vi "Main.vi"() -> ()   [LabVIEW 2019]
uses:
  States/TaskType.ctl
  States/Main_States.ctl
  States/Hand.ctl
  States/ROM_States.ctl
  Shared VIs/ClusterType/RobotStateType.ctl
  <vilib>/myRIO/Common/Instrument Driver Framework/myRIO v1.0/Encoder/typedefs/Encoder Signal Mode.ctl
  Shared VIs/Messages/NewPatientNotifierArgs.ctl
  Shared VIs/ModelSpecific/ETHMikeModel.ctl
  Shared VIs/ModelSpecific/ReadOnlyGlobalActions.ctl
  <vilib>/myRIO/Instrument Drivers/Onboard IO/AI/typedefs/AI Reference.ctl
  <vilib>/myRIO/Common/Instrument Driver Framework/Utilities/typedefs/myRIO Generic Hardware Reference.ctl
  <vilib>/myRIO/Common/Instrument Driver Framework/Utilities/typedefs/Hardware Version Enum.ctl
  <vilib>/myRIO/Common/Instrument Driver Framework/Utilities/typedefs/myRIO v1.0 Reference.ctl
  <vilib>/myRIO/Common/Instrument Driver Framework/Utilities/typedefs/Generic FPGA Reference.ctl
  <vilib>/myRIO/Common/Instrument Driver Framework/myRIO v1.0/AI/typedefs/AI Channels List.ctl
  <vilib>/myRIO/Common/Instrument Driver Framework/myRIO v1.0/AI/typedefs/AI Channels Enum.ctl
  <vilib>/myRIO/Common/Instrument Driver Framework/Utilities/typedefs/Analog Scaling Constants List.ctl
  <vilib>/myRIO/Common/Instrument Driver Framework/Utilities/typedefs/Analog Scaling Constants.ctl
  <vilib>/userDefined/High Color/nirio_resource_hc.ctl
  <vilib>/myRIO/Instrument Drivers/Onboard IO/AO/typedefs/AO Reference.ctl
  <vilib>/myRIO/Common/Instrument Driver Framework/myRIO v1.0/AO/typedefs/AO Channels List.ctl
  <vilib>/myRIO/Common/Instrument Driver Framework/myRIO v1.0/AO/typedefs/AO Channels Enum.ctl
  Shared VIs/ClusterType/TaskInfoType.ctl
  <vilib>/Platform/TimedLoop/XDataNode/timing_clust.ctl
  <vilib>/Platform/TimedLoop/XDataNode/nitl_modes.ctl
  <vilib>/Platform/TimedLoop/XDataNode/wakeup.ctl
  Shared VIs/Messages/UdpGlobalActions.ctl
  Shared VIs/TypeDef_TDMS_States.ctl
  Shared VIs/Messages/MsgHeader.ctl
  Shared VIs/Messages/PatientSelectMsg.ctl
  Shared VIs/Messages/CommandMsg.ctl
  Shared VIs/Messages/BackendInfoMsg.ctl
  <vilib>/myRIO/Common/Instrument Driver Framework/myRIO v1.0/AI/vis/myRIO v1.1 Open AI.vi
  <vilib>/myRIO/Common/Instrument Driver Framework/myRIO v1.0/AO/vis/myRIO v1.1 Open AO.vi
  <vilib>/myRIO/Common/Instrument Driver Framework/Utilities/vis/Validate Channels.vi
  <vilib>/myRIO/Common/Instrument Driver Framework/myRIO v1.0/AI/vis/myRIO v1.0 Reserve AI.vi
  <vilib>/myRIO/Common/Instrument Driver Framework/myRIO v1.0/AO/vis/myRIO v1.0 Reserve AO.vi
  <vilib>/myRIO/Common/Instrument Driver Framework/myRIO v1.0/AI/vis/myRIO v1.0 Close AI.vi
  <vilib>/myRIO/Common/Instrument Driver Framework/myRIO v1.0/Encoder/vis/myRIO v1.0 Close Encoder.vi
  <vilib>/myRIO/Common/Instrument Driver Framework/myRIO v1.0/AO/vis/myRIO v1.0 Close AO.vi
  <vilib>/myRIO/Common/Instrument Driver Framework/myRIO v1.0/AI/vis/myRIO v1.0 Build MUX Configuration AI.vi
  <vilib>/myRIO/Common/Instrument Driver Framework/myRIO v1.0/Resource Manager/vis/myRIO v1.0 Reserve Channel List.vi
  <vilib>/myRIO/Common/Instrument Driver Framework/myRIO v1.0/AO/vis/myRIO v1.0 Build MUX Configuration AO.vi
  <vilib>/myRIO/Common/Instrument Driver Framework/myRIO v1.0/AI/vis/myRIO v1.0 Unreserve AI.vi
  <vilib>/myRIO/Common/Instrument Driver Framework/myRIO v1.0/Encoder/vis/myRIO v1.0 Unreserve Encoder.vi
  <vilib>/myRIO/Common/Instrument Driver Framework/myRIO v1.0/AO/vis/myRIO v1.0 Unreserve AO.vi
  <vilib>/myRIO/Common/Instrument Driver Framework/myRIO v1.0/Resource Manager/vis/myRIO v1.0 Reserve Channel.vi
  <vilib>/myRIO/Common/Instrument Driver Framework/myRIO v1.0/Resource Manager/vis/myRIO v1.0 Unreserve Channel.vi
  <vilib>/myRIO/Common/Instrument Driver Framework/myRIO v1.0/Resource Manager/vis/myRIO v1.0 Unreserve Channel List.vi
  <vilib>/myRIO/Common/Instrument Driver Framework/myRIO v1.0/Encoder/vis/myRIO v1.0 Build MUX Configuration Encoder.vi
  <vilib>/myRIO/Common/Instrument Driver Framework/myRIO v1.0/Resource Manager/vis/myRIO v1.0 Build Mutex Name.vi
  <vilib>/myRIO/Common/Instrument Driver Framework/myRIO v1.0/Resource Manager/vis/myRIO v1.0 Create Configuration List.vi
  <vilib>/Utility/VariantDataType/GetNumericInfo.vi
  <vilib>/Utility/error.llb/Error Cluster From Error Code.vi
  <vilib>/myRIO/Common/Instrument Driver Framework/myRIO v1.0/myRIO v1.1 Open.vi
  <vilib>/myRIO/Common/Instrument Driver Framework/myRIO v1.0/AO/vis/myRIO v1.0 Get Scaling Constants AO.vi
  <vilib>/myRIO/Common/Instrument Driver Framework/Utilities/vis/IO Manager.vi
  <vilib>/myRIO/Common/Instrument Driver Framework/Utilities/vis/Configuration Manager.vi
  <vilib>/myRIO/Common/Instrument Driver Framework/myRIO v1.0/myRIO v1.0 Close.vi
  <vilib>/myRIO/Common/Instrument Driver Framework/myRIO v1.0/AO/vis/myRIO v1.0 Write AO.vi
  <vilib>/myRIO/Common/Instrument Driver Framework/myRIO v1.0/AI/vis/myRIO v1.0 Get Scaling Constants AI.vi
  <vilib>/functionblocks/Counter/Elapsed Timer/Elapsed Timer.vi
  <vilib>/myRIO/Common/Instrument Driver Framework/myRIO v1.0/Encoder/vis/myRIO v1.0 Enable Encoder.vi
  <vilib>/myRIO/Common/Instrument Driver Framework/myRIO v1.0/Encoder/vis/myRIO v1.0 Shutdown Encoder.vi
  <vilib>/myRIO/Common/Instrument Driver Framework/myRIO v1.0/Resource Manager/vis/myRIO v1.0 Configure IO.vi
  <vilib>/myRIO/Instrument Drivers/Onboard IO/AO/vis/myRIO AO Open.xnode
  <vilib>/myRIO/Instrument Drivers/Onboard IO/AI/vis/myRIO AI Open.xnode
  <vilib>/Platform/TimedLoop/XDataNode/XDataNode.xnode
  <vilib>/functionblocks/FB Core/FB Core.xnode
  <vilib>/myRIO/Instrument Drivers/Onboard IO/AO/AO.lvlib
  <vilib>/Platform/TimedLoop/XDataNode/XDNodeRunTimeDep.lvlib
  <vilib>/myRIO/Instrument Drivers/Onboard IO/Encoder/Encoder.lvlib
  <vilib>/myRIO/Instrument Drivers/Onboard IO/AI/AI.lvlib
  <vilib>/functionblocks/NI_FunctionBlock Libraries.lvlib
  <vilib>/addons/control/pid/NI_PID_pid.lvlib
  <vilib>/ptbypt/NI_PtbyPt.lvlib
panel:
  out "start value":dbl
  out "Haptic Bump Force Frontend [N]":dbl
  out "difference at start":dbl
  out "Direction":i32
  out "Haptic Bump Force [N]":dbl format="%#_13g"
  out "Plateau length [deg]":dbl
  out "Ramp length [deg]":dbl=4.0 format="%#_13g"
  out "Starting Position Frontend [deg]":dbl
  out "Target Position Frontend [deg]":dbl
  out "RobotState":T1
  out "SkipSignal":bool
  out "Force_calib_value":dbl
  out "Velocity_calib_value":dbl
  out "LogFileOpen":bool
  out "Phase Trial Count":i16
  out "Error which lead\nto TCP close":errorcluster
  out "TCP Error":errorcluster
  out "UDP Error":errorcluster
  in  "stop":bool
  out "SelectedHand":T2
  out "Connected":bool
  out "Remote IP":u32 format="%x"
  out "StopRequested":bool
  in  "TCP Server Port":u16=6662
  in  "UDP Destination Port":u16=6661
  out "DateTime":string
  out "SubjectNr":string
  out "StopSignal":bool
  out "RestartSignal":bool
  out "StartSignal":bool
  out "FrontendStartedSignal":bool
  out "Flexion":bool
  out "TaskFinished":bool
  out "ROM State":T3=enum."Passive"
  out "LeftHand":bool
  out "Machine State":T4=enum."StartTrial"
  out "MovingToTarget":bool=TRUE
  out "ROM max":dbl
  out "ROM min":dbl
  out "Zero Position":dbl
  out "Largest USB Partition Path":path
  out "Trial Nr":i16
  out "Starting position":dbl
  out "Target Array":dbl[](array[numeric])
  out "TaskType":T5
  out "Current Setpoint [A]":dbl
  out "Finished late?":bool
  out "Target state?":bool
  out "Target Position [deg]":dbl
  # "Frontend Connection"
  # "Command Signals"
  # "Robot State"
  # "Patient Data"
  # "Task State"
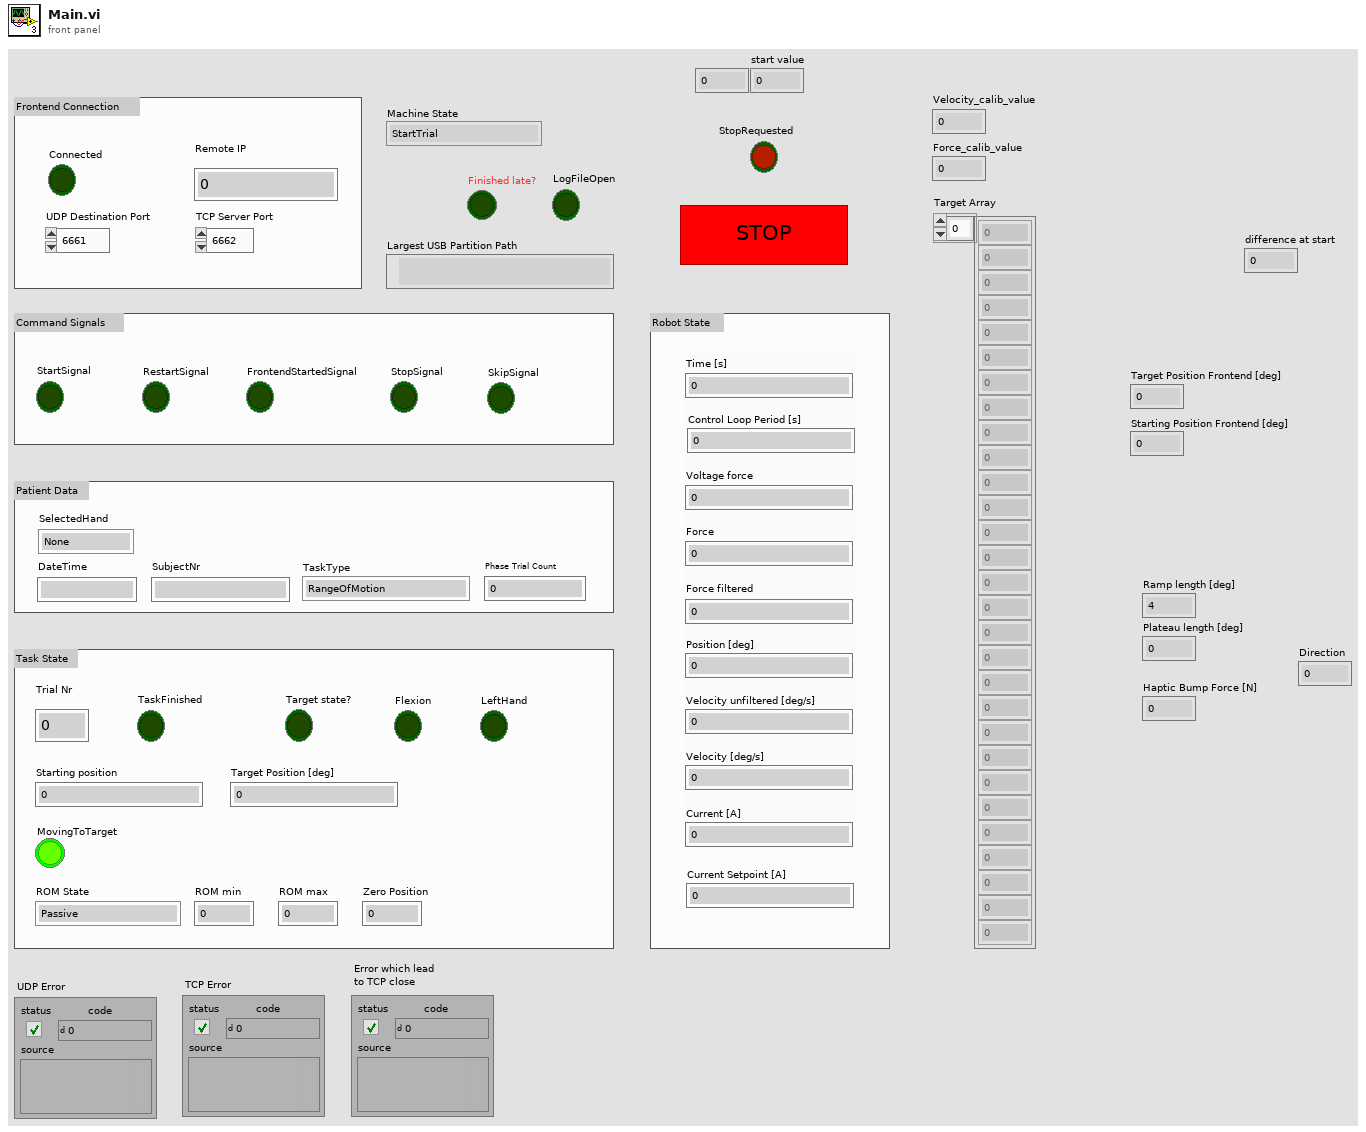
[diagram p1: front panel]
types:
  T1 = typedef "RobotStateType.ctl" = cluster{"Time [s]":dbl, "Voltage force":dbl, "Force":dbl, "Force filtered":dbl, "Position [deg]":dbl, "Velocity unfiltered [deg/s]":dbl, "Velocity [deg/s]":dbl, "Current [A]":dbl, "Control Loop Period [s]":dbl}
  T2 = typedef "Hand.ctl" = enum8{"None", "Left", "Right"}
  T3 = typedef "ROM_States.ctl" = enum8{"Active", "Passive", "AutomaticPassive"}
  T4 = typedef "Main_States.ctl" = enum16{"Hand choice", "StartTask", "StartTrial", "Show target", "Resetting", "WaitingForRestart"}
  T5 = typedef "TaskType.ctl" = enum8{"RangeOfMotion", "Force", "Motor", "Sensorimotor", "PositionMatching", "PreciseReaching", "PassiveMatching", "ActiveMatching", "TeachAndReproduce", "HapticBump"}
  T6 = typedef "NewPatientNotifierArgs.ctl" = cluster{"Left":bool, "Mode":T5, "Name":string, "Timestamp":string, "StudyName":string}
  T7 = cluster{"read mode":enum16{"polling", "blocking"}, "write mode":enum16{"polling", "blocking"}}
  T8 = typedef "nirio_resource_hc.ctl" = tag
  T9 = typedef "Hardware Version Enum.ctl" = enum16{"Unknown", "myRIO-1900", "myRIO-1950", "roboRIO", "NI ELVIS RIO CM", "ELVIS III"}
  T10 = typedef "TypeDef_TDMS_States.ctl" = enum16{"WaitingForCreate", "Create", "Buffering", "Flushing", "Write", "Close"}
  T11 = enum16{"open", "open or create", "create or replace", "create", "open (read-only)"}
  T12 = typedef "XDNodeRunTimeDep.lvlib/timing_clust.ctl" = cluster{"Expected End [f-1]":u64, "Actual End [f-1]":u64, "Finished Late? [f-1]":bool, "Expected End [i-1]":u64, "Actual End [i-1]":u64, "Finished Late? [i-1]":bool, "Expected Start [i]":u64, "Actual Start [i]":u64, "Expected Start [f]":u64, "Actual Start [f]":u64, "Source Name":string, "Structure Name":string, "Period":i64, "Deadline":i64, "Offset":i64, "Start":i64, "Priority":i32, "Timeout":i32, "Mode":T13, "Wakeup Reason":T14, "Error":errorcluster, "Source Type":string, "Secondary Source Type":string, "Global End Time":u64, "Global Start Time":u64, "Frame Duration":u64, "Iteration Duration":u64, "Assigned CPU":i32, "I/O Scan Engine Mode":u32}
  T13 = typedef "XDNodeRunTimeDep.lvlib/nitl_modes.ctl" = enum32{"No Change", "Process missed periods, maintain original phase", "Discard missed periods, maintain original phase", "Process missed periods, ignore original phase", "Discard missed periods, ignore original phase"}
  T14 = typedef "XDNodeRunTimeDep.lvlib/wakeup.ctl" = enum32{"Normal", "Aborted", "Asynchronous wakeup", "Timing source error", "Timed loop error", "Timeout"}
  T15 = enum8{"Invalid", "PatientSelect", "Command", "Skip", "BackendInfoReq", "UnknownOp (Must be Last)"}
  T16 = typedef "MsgHeader.ctl" = cluster{"MsgType [0]":u8, "MsgLen [1:2]":u16}
  T17 = typedef "PatientSelectMsg.ctl" = cluster{"LeftHand":bool, "AssessmentMode":u8, "SubjectNr":string, "DateTime":string, "PhaseTrialCount":i32, "StudyName":string}
  T18 = typedef "CommandMsg.ctl" = cluster{"EmergencyStop":bool, "Start":bool, "Restart":bool, "FrontendStarted":bool, "Close":bool, "StartingPosition":sgl, "TargetPosition":sgl, "HapticBumpForce":dbl}
  T19 = typedef "BackendInfoMsg.ctl" = cluster{"ProtocolVersion":u16, "DataPath":string}
  T20 = typedef "UdpGlobalActions.ctl" = enum16{"Read", "Write"}
  T21 = typedef "ReadOnlyGlobalActions.ctl" = enum16{"Initialize", "Read", "Write"}
  T22 = typedef "ETHMikeModel.ctl" = enum16{"ETH Mike #1", "ETH Mike #2", "ETH Mike #3", "ETH Mike #4", "ETH MIKE #5"}
  T23 = typedef "Encoder Signal Mode.ctl" = enum16{"Quadrature phase signal", "Step and direction signal"}
  T24 = typedef "AO.lvlib/AO Reference.ctl" = cluster{"myRIO Reference":T25, "AO Channel List":T28, "AO Scaling Constant List":T30}
  T25 = typedef "myRIO Generic Hardware Reference.ctl" = cluster{"myRIO Model":T9, "myRIO Hardware Reference":T26}
  T26 = typedef "myRIO v1.0 Reference.ctl" = cluster{"Generic FPGA Reference":T27, "Allow multiple opens":bool}
  T27 = typedef "Generic FPGA Reference.ctl" = refnum<k20>
  T28 = typedef "AO Channels List.ctl" = T29[]
  T29 = typedef "AO Channels Enum.ctl" = enum16{"Not Connected", "AudioOut/Left", "AudioOut/Right", "C/AO0", "C/AO1", "A/AO0", "A/AO1", "B/AO0", "B/AO1"}
  T30 = typedef "Analog Scaling Constants List.ctl" = T31[]
  T31 = typedef "Analog Scaling Constants.ctl" = cluster{"LSB Weight (Volts)":dbl, "Offset (Volts)":dbl, "Signed?":bool}
  T32 = typedef "Encoder.lvlib/Encoder Reference.ctl" = cluster{"myRIO Reference":T25, "Encoder Channels Enum":T33}
  T33 = typedef "Encoder Channels Enum.ctl" = enum16{"Not Connected", "C/ENC0", "C/ENC1", "A/ENC", "A/ENC0", "A/ENC1", "A/ENC2", "A/ENC3", "A/ENC4", "A/ENC5", "A/ENC6", "A/ENC7", "A/ENC8", "A/ENC9", "B/ENC", "B/ENC0", "B/ENC1", "B/ENC2", "B/ENC3", "B/ENC4", "B/ENC5", "B/ENC6", "B/ENC7", "B/ENC8", "B/ENC9", "DIO/ENC0", "DIO/ENC1", "DIO/ENC2", "DIO/ENC3", "DIO/ENC4"}
  T34 = typedef "AI.lvlib/AI Reference.ctl" = cluster{"myRIO Reference":T25, "AI Channels List":T35, "AI Scaling Constants List":T30}
  T35 = typedef "AI Channels List.ctl" = T36[]
  T36 = typedef "AI Channels Enum.ctl" = enum16{"Not Connected", "AudioIn/Left", "AudioIn/Right", "C/AI0", "C/AI1", "A/AI0", "A/AI1", "A/AI2", "A/AI3", "A/AI4", "A/AI5", "A/AI6", "A/AI7", "B/AI0", "B/AI1", "B/AI2", "B/AI3", "B/AI4", "B/AI5", "B/AI6", "B/AI7", "AI/AI0", "AI/AI1", "AI/AI2", "AI/AI3", "A/AI0 (DIFF)", "A/AI1 (DIFF)", "A/AI2 (DIFF)", "A/AI3 (DIFF)", "B/AI0 (DIFF)", "B/AI1 (DIFF)", "B/AI2 (DIFF)", "B/AI3 (DIFF)"}
  T37 = cluster{"Encoder":T32, "Tachometer":T34, "Motor Current Monitor":T34, "Force Sensor":T34}
  T38 = typedef "LVAllMonitorsDisplayTypeDef.ctl" = cluster{"Bounds":cluster{"Left":i16, "Top":i16, "Right":i16, "Bottom":i16}, "Depth":i16}[]
  T39 = cluster{"Bounds":cluster{"Left":i16, "Top":i16, "Right":i16, "Bottom":i16}, "Depth":i16}
  T40 = cluster{"Left":i16, "Top":i16, "Right":i16, "Bottom":i16}
  T41 = typedef "TaskInfoType.ctl" = cluster{"Task Type":T5, "Phase Trial Count":i16, "Left Hand":bool}
  T42 = enum16{"Standard", "Buffered", "CRLF", "Immediate"}
  T43 = typedef "UDPRobotState.ctl" = cluster{"Counter":u32, "Time":sgl, "Position":sgl, "StartingPosition":sgl, "TargetPosition":sgl, "Force":sgl, "TrialNr":u8, "RomState":u8, "TargetState":bool, "Finished":bool, "Flexion":bool}
  T44 = typedef "PID_Settings.ctl" = cluster{"Gains":T45, "Non-linear gain":T46, "D-Part variable":T48, "Velocity estimate dy/dt":T49, "Anti reset windup":bool, "I-Part error band":dbl, "Output range":T50}
  T45 = typedef "Gains.ctl" = cluster{"K(e)":dbl, "Kp":dbl, "Ki":dbl, "Kd":dbl}
  T46 = typedef "NonLinearGainParams.ctl" = cluster{"Non-linear gain P":T47, "Non-linear gain I":T47, "Non-linear gain D":T47}
  T47 = typedef "NonLinearGain.ctl" = enum16{"exponential", "quadratic", "off"}
  T48 = typedef "DPartVariable.ctl" = enum16{"error", "process variable"}
  T49 = typedef "VelocityEstimate.ctl" = enum16{"derivative", "external"}
  T50 = typedef "OutputRange.ctl" = cluster{"output high":dbl, "output low":dbl}
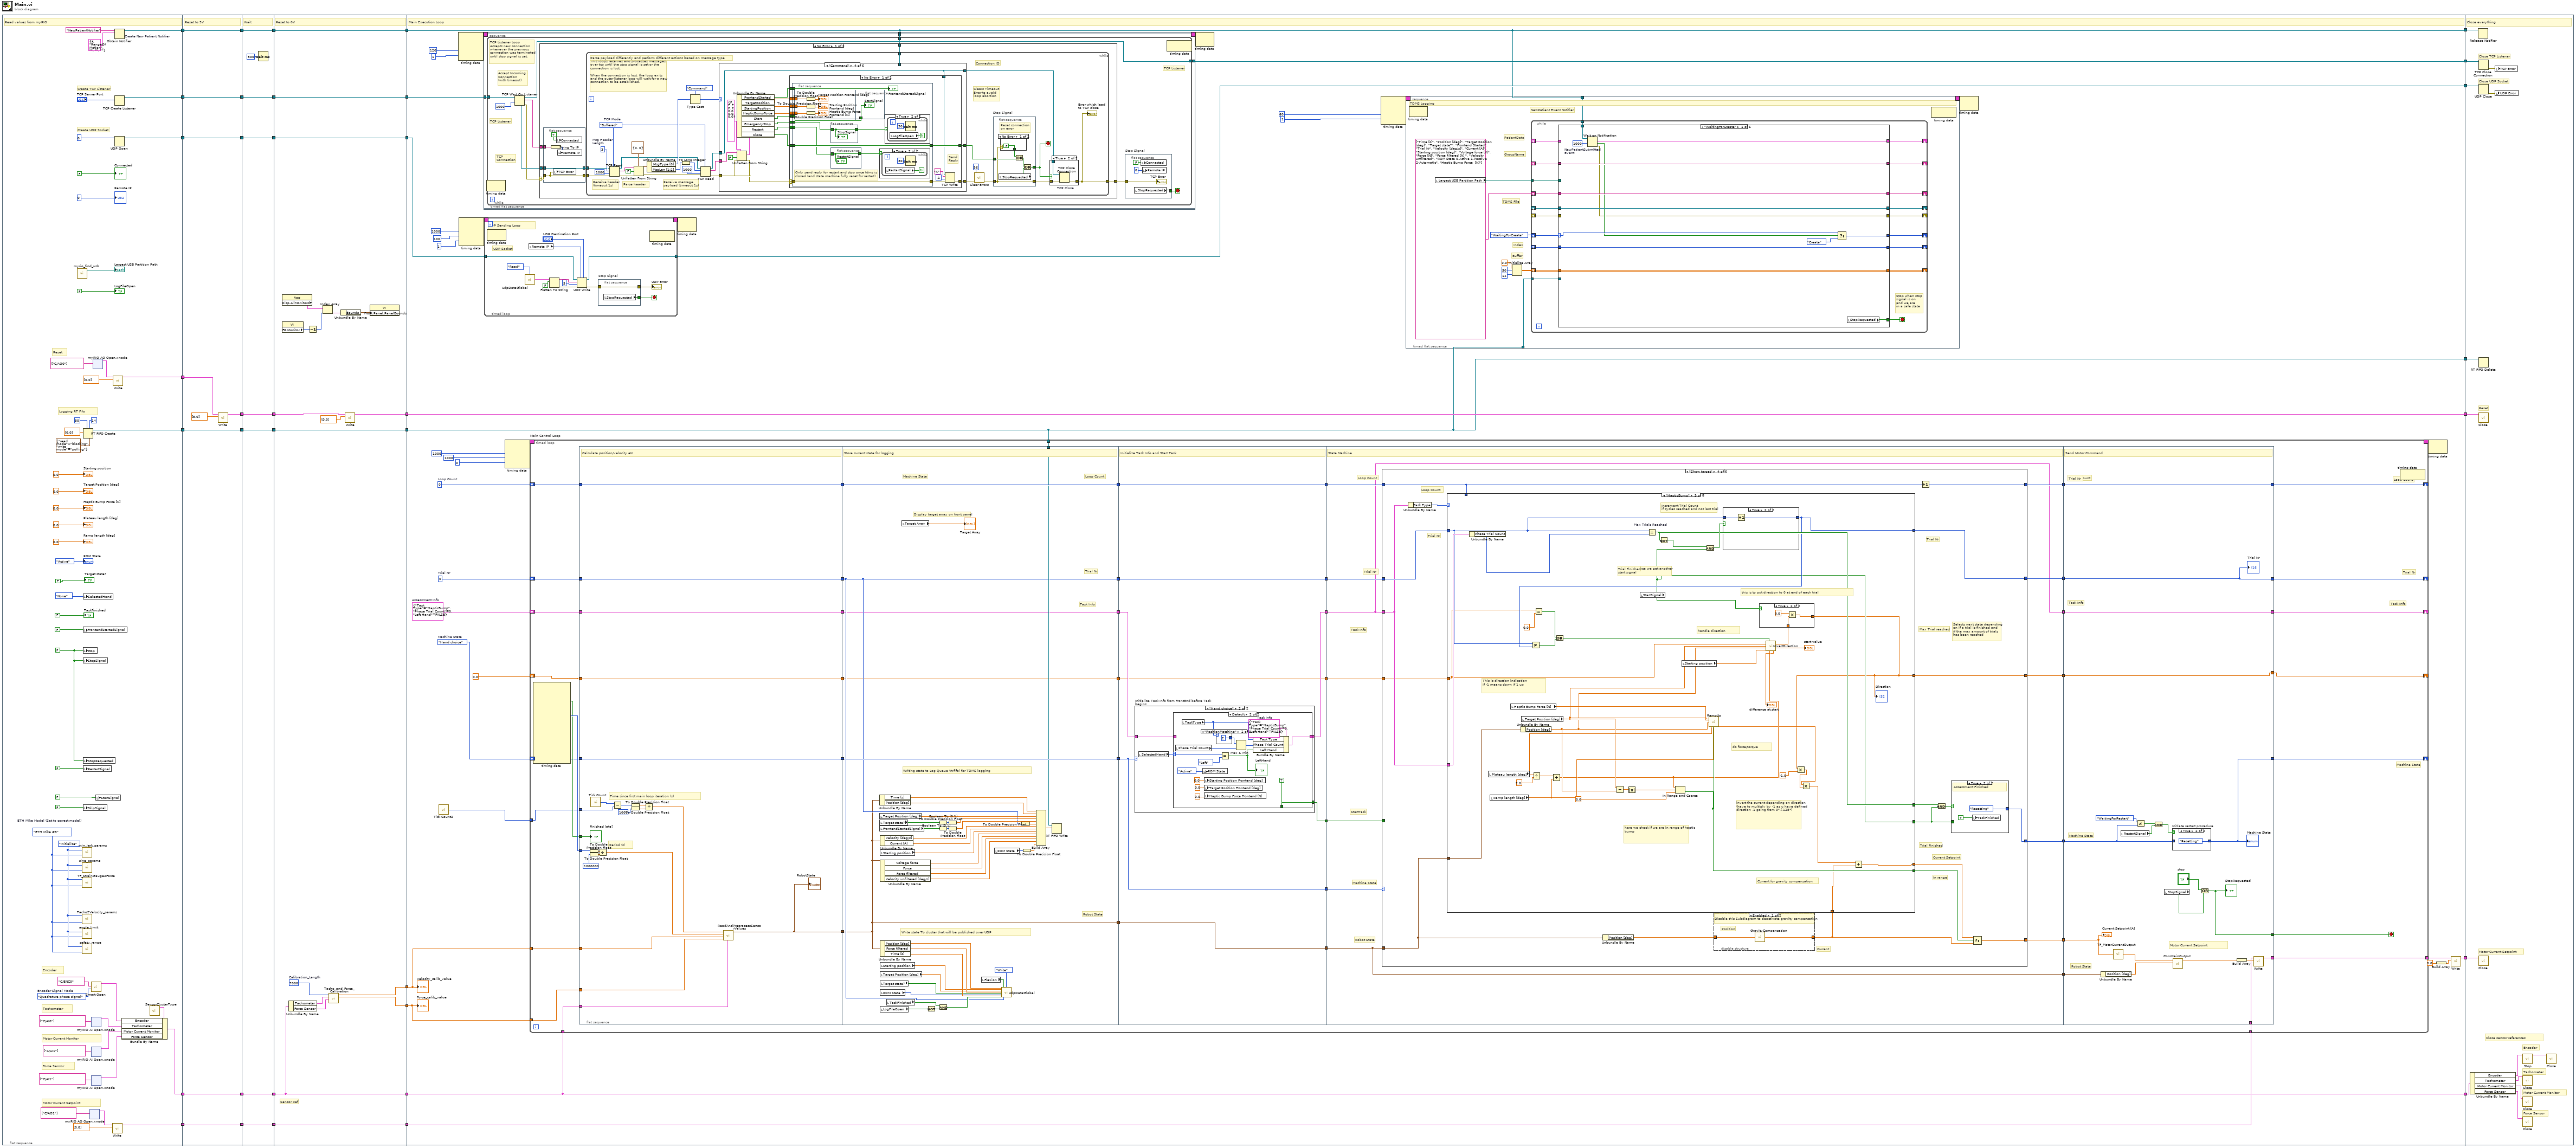
[diagram p0: block diagram]
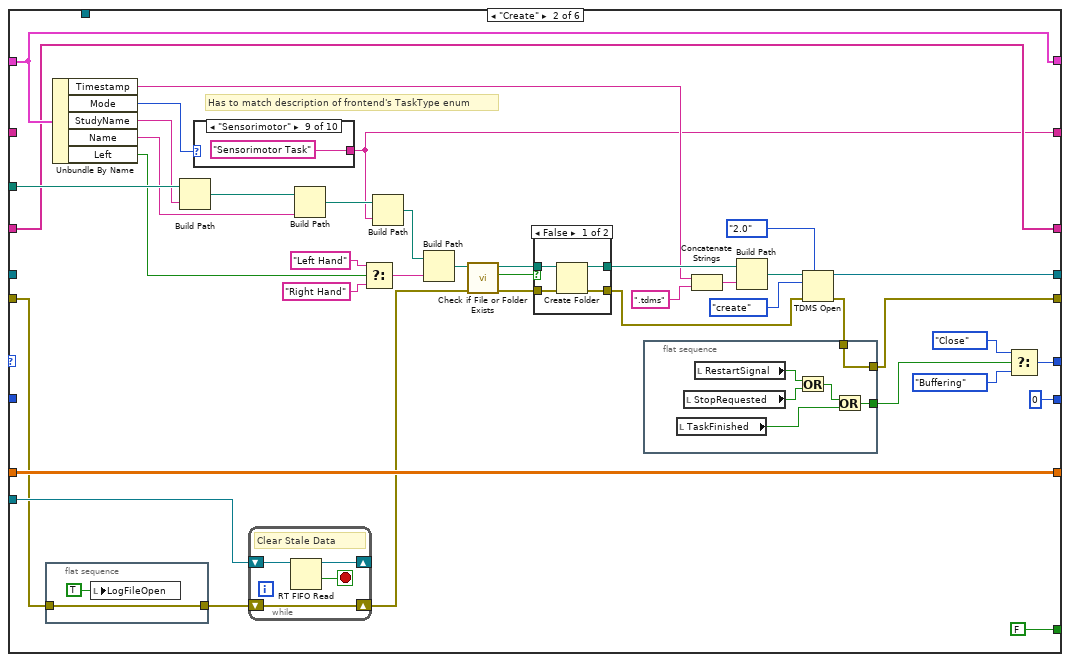
[diagram p2: hidden frame]
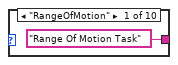
[diagram p4: hidden frame]
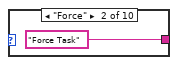
[diagram p5: hidden frame]
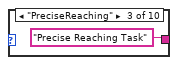
[diagram p6: hidden frame]
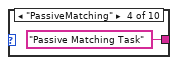
[diagram p7: hidden frame]
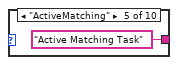
[diagram p8: hidden frame]
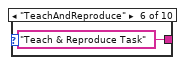
[diagram p9: hidden frame]
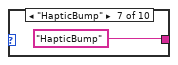
[diagram p10: hidden frame]
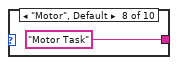
[diagram p11: hidden frame]
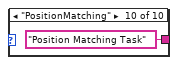
[diagram p12: hidden frame]
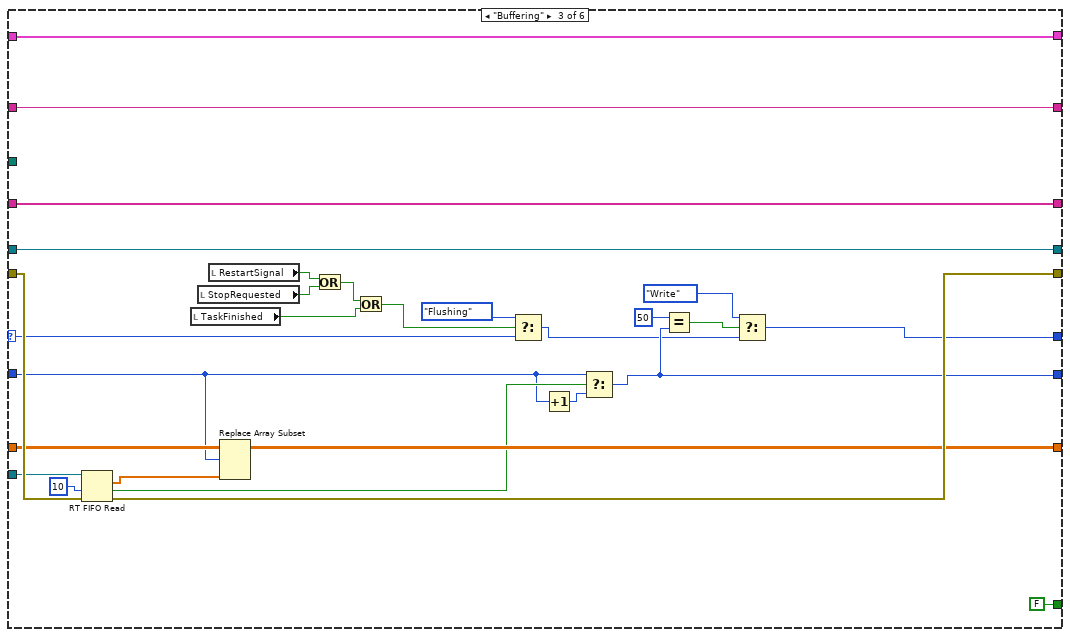
[diagram p13: hidden frame]
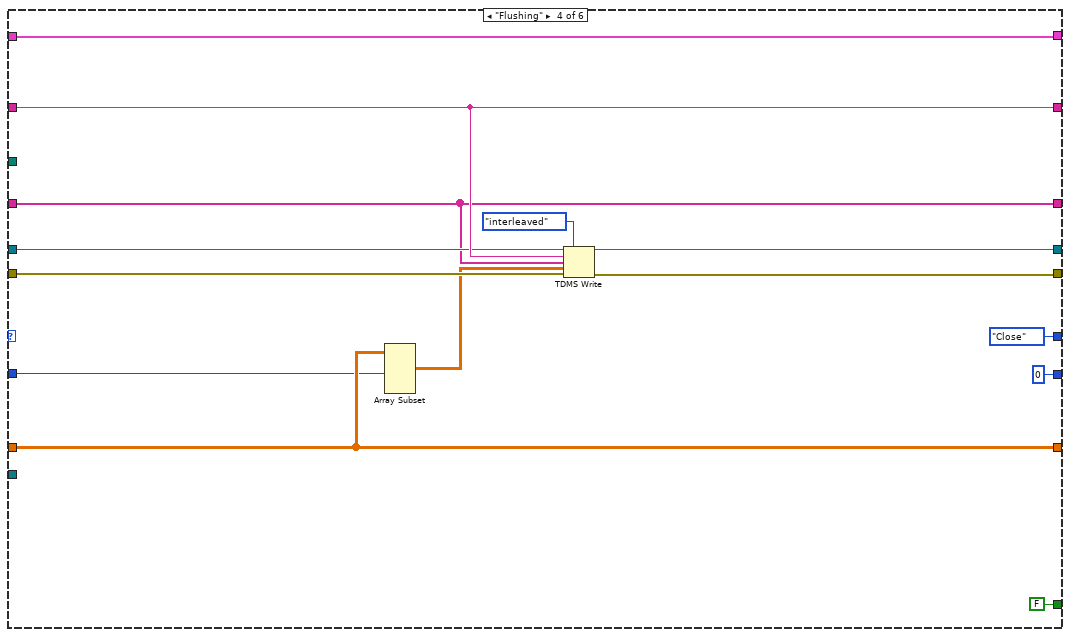
[diagram p14: hidden frame]
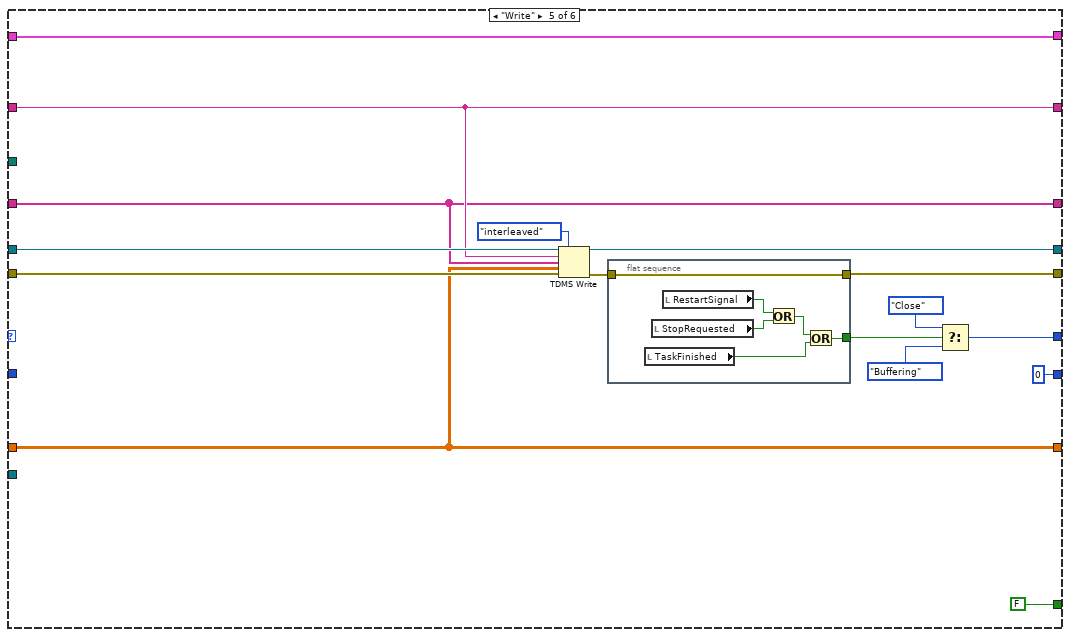
[diagram p15: hidden frame]
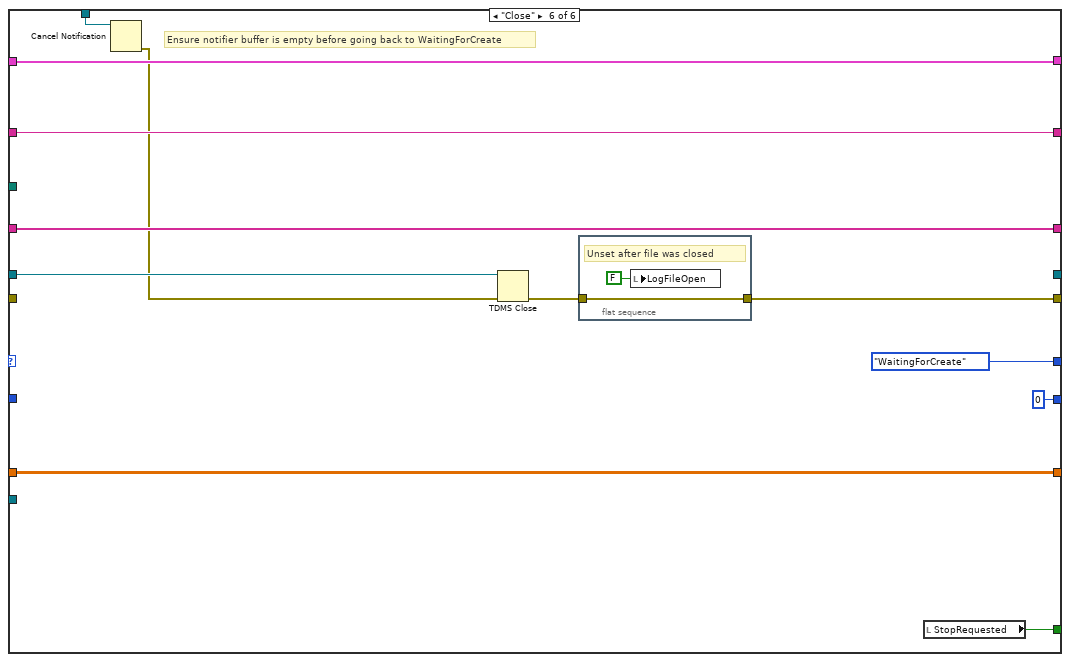
[diagram p16: hidden frame]
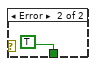
[diagram p18: hidden frame]
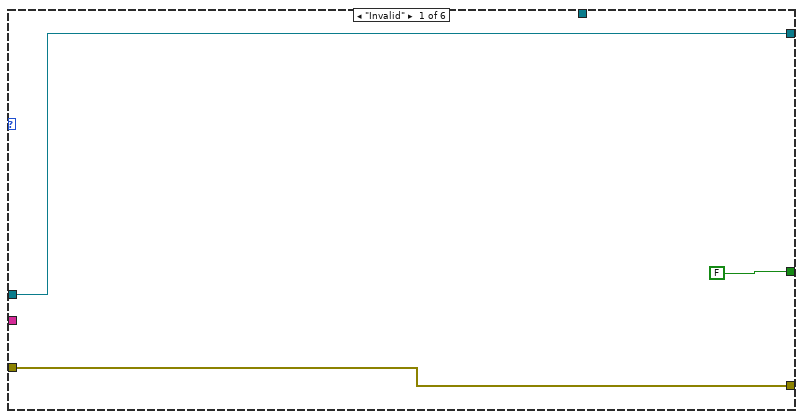
[diagram p19: hidden frame]
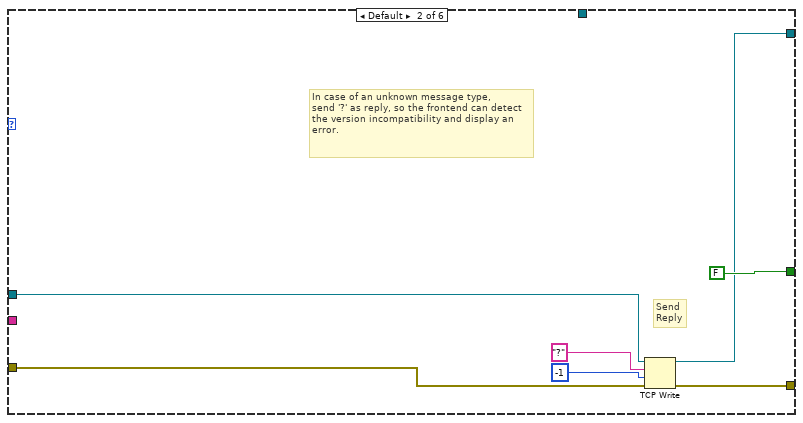
[diagram p20: hidden frame]
diagram:
  n1 = flat-sequence {
    tunnel: [w78] -> w37
    tunnel: [w69] -> w28
    tunnel: [w67] -> w24
    tunnel: [w56] -> w18
    tunnel: [w55] -> w14
    tunnel: [w42] -> w7
    tunnel: [w41] -> w1
    tunnel: w37 -> [w186]
    tunnel: [w185] -> w36
    tunnel: [w184] -> w29
    tunnel: w28 -> [w184]
    tunnel: [w183] -> w25
    tunnel: w24 -> [w183]
    tunnel: [w182] -> w19
    tunnel: w18 -> [w182]
    tunnel: [w181] -> w15
    tunnel: w14 -> [w181]
    tunnel: [w180] -> w8
    tunnel: w7 -> [w180]
    tunnel: [w179] -> w2
    tunnel: w1 -> [w179]
    tunnel: w36 -> [w194]
    tunnel: [w194] -> w35
    tunnel: [w193] -> w30
    tunnel: w29 -> [w193]
    tunnel: [w192] -> w26
    tunnel: w25 -> [w192]
    tunnel: [w191] -> w20
    tunnel: w19 -> [w191]
    tunnel: [w190] -> w16
    tunnel: w15 -> [w190]
    tunnel: [w189] -> w9
    tunnel: w8 -> [w189]
    tunnel: [w188] -> w3
    tunnel: w2 -> [w188]
    tunnel: w35 -> [w213]
    tunnel: [w212] -> w34
    tunnel: [w206] -> w31
    tunnel: w30 -> [w206]
    tunnel: w26 -> [w205]
    tunnel: [w205] -> w23
    tunnel: [w204] -> w21
    tunnel: w20 -> [w204]
    tunnel: [w203] -> w17
    tunnel: w16 -> [w203]
    tunnel: [w201] -> w11
    tunnel: [w200] -> w10
    tunnel: w9 -> [w197]
    tunnel: [w197] -> w6
    tunnel: [w196] -> w4
    tunnel: w3 -> [w196]
    tunnel: w34 -> [w251]
    tunnel: [w225] -> w33
    tunnel: [w251] -> w32
    tunnel: w31 -> [w244]
    tunnel: [w234] -> w27
    tunnel: w23 -> [w243]
    tunnel: [w233] -> w22
    tunnel: w21 -> [w219]
    tunnel: w17 -> [w227]
    tunnel: [w227] -> w13
    tunnel: [w219] -> w12
    tunnel: w11 -> [w216]
    tunnel: w10 -> [w222]
    tunnel: w6 -> [w221]
    tunnel: [w221] -> w5
    tunnel: w4 -> [w217]
    tunnel: w33 -> [w1526]
    tunnel: w32 -> [w1533]
    tunnel: w27 -> [w1532]
    tunnel: w22 -> [w1531]
    tunnel: w13 -> [w1528]
    tunnel: w12 -> [w1527]
    tunnel: w5 -> [w1525]
    frame #0 {
      w49 = ReadOnlyGlobalActions."Initialize" ("Action (Read)")
      w48 = ETHMikeModel."ETH Mike #3"  # ETH Mike Model (Set to correct model)
      w63 = FALSE ("stop")
      w84 = Encoder_Signal_Mode."Quadrature phase signal"  # Encoder Signal Mode
      # "Logging RT Fifo"
      # "Create TCP Listener"
      # "Create UDP Socket"
      # "Force Sensor"
      # "Tachometer"
      # "Motor Current Monitor"
      # "Motor Current Setpoint"
      # "Reset"
      # "Encoder"
      # "Read values from myRIO"
      n2 = call "myrio_find_usb.vi"() -> ("Largest USB Partition Path"=→"Largest USB Partition Path":path)  [unwired: 9 in, 2 out]
      n3 = call "min_jerk_params.vi"("Action (Read)"=w49, "ETH Mike Model"=w48) -> ()  [unwired: 17 in, 1 out]
      n4 = call "sine_params.vi"("Action (Read)"=w49, "ETH Mike Model"=w48) -> ()  [unwired: 17 in, 1 out]
      n5 = call "TF_StrainGauge2Force.vi"("Action (Read)"=w49, "ETH Mike Model"=w48) -> ()  [unwired: 3 in, 1 out]
      n6 = call "Tacho2Velocity_params.vi"("Action (Read)"=w49, "ETH Mike Model"=w48) -> ()  [unwired: 3 in, 1 out]
      n7 = call "angle_limit.vi"("ETH Mike Model"=w48, "Action (Read)"=w49) -> ()  [unwired: 1 out]
      n8 = call "safety_range.vi"("ETH Mike Model"=w48, "Action (Read)"=w49) -> ()  [unwired: 1 out]
      n9 = RT FIFO Create(1:dbl[] [0.0] ("Values"), 4:u32 50 ("size (10)"), 6:u32 14 ("elements in array (1)"), 7:T7 {"read mode"=enum."blocking", "write mode"=enum."polling"} ("r/w modes (polling,polling)")) -> (8:w56:refnum<k33>)  [unwired: 4 in, 2 out]
      n10 = local write "SelectedHand"(Hand."None" ("Enum")) -> ()
      n11 = local write "FrontendStartedSignal"(FALSE) -> ()
      n12 = local write "stop"(w63) -> ()
      n13 = local write "StopSignal"(w63) -> ()
      n14 = local write "StopRequested"(w63) -> ()
      n15 = local write "RestartSignal"(FALSE ("Restart")) -> ()
      n16 = local write "SkipSignal"(FALSE ("StartSignal")) -> ()
      n17 = xnode "myRIO AO Open.xnode"("Channel Names"=tag[] ["C/AO1"]) -> ("AO Ref Out"=w82:T24)  [unwired: 2 in, 1 out]
      n18 = call <vilib>:"Smart Open.vi"("Encoder Signal Mode"=w84, "Channel Name"=tag "C/ENC0") -> ("Encoder Ref Out"=w46:T32)  [unwired: 8 in, 1 out]
      n19 = xnode "myRIO AI Open.xnode"("Channel Names"=tag[] ["C/AI0"]) -> ("AI Ref Out"=w45:T34)  [unwired: 2 in, 1 out]
      n20 = xnode "myRIO AI Open.xnode"("Channel Names"=tag[] ["A/AI1"]) -> ("AI Ref Out"=w44:T34)  [unwired: 2 in, 1 out]
      n21 = xnode "myRIO AI Open.xnode"("Channel Names"=tag[] ["C/AI1"]) -> ("AI Ref Out"=w43:T34)  [unwired: 2 in, 1 out]
      n22 = xnode "myRIO AO Open.xnode"("Channel Names"=tag[] ["C/AO0"]) -> ("AO Ref Out"=w87:T24)  [unwired: 2 in, 1 out]
      n23 = local write "StartSignal"(FALSE ("StartSignal")) -> ()
      n24 = call <vilib>:"Write.vi"("Values"=dbl[] [0.0], "AO Ref In"=w82) -> ("AO Ref Out"=w41:T24)  [unwired: 7 in, 1 out]
      n25 = call <vilib>:"Write.vi"("Values"=dbl[] [0.0], "AO Ref In"=w87) -> ("AO Ref Out"=w78:T24)  [unwired: 7 in, 1 out]
      n26 = Obtain Notifier "Create New Patient Notifier"(name (unnamed)="NewPatientNotifier", notification data type=T6 {"Left"=FALSE, "Mode"=enum."RangeOfMotion", "Name"="", "Timestamp"="", "StudyName"=""}) -> (notifier out=w55:refnum<notifier>)  [unwired: 2 in, 2 out]
      n27 = TCP Create Listener(10:"TCP Server Port") -> (3:w67:refnum<k5>)  [unwired: 4 in, 2 out]
      n28 = UDP Open(11:u16 0) -> (port=w69:refnum<k16>)  [unwired: 4 in, 2 out]
      n29 = call "SensorClusterType.vi"() -> ("Cluster"=w47:T37)  [unwired: 11 in]
      n30 = Bundle By Name(cluster=w47, "Encoder"=w46, "Tachometer"=w45, "Motor Current Monitor"=w44, "Force Sensor"=w43) -> (w42:T37)
      "Target state?" <- FALSE ("Target state?")
      "Target Position [deg]" <- 0.0 ("Target Position [deg]")
      "ROM State" <- ROM_States."Active" ("Enum")
      "Connected" <- FALSE
      "Remote IP" <- u32 0
      "LogFileOpen" <- FALSE ("LogFileOpen")
      "TaskFinished" <- FALSE ("AssessmentFinished")
      "Starting position" <- 0.0 ("Starting position")
      "Ramp length [deg]" <- 0.0
      "Plateau length [deg]" <- 0.0 ("Target Position [deg]")
      "Haptic Bump Force [N]" <- 0.0
    }
    frame #1 {
      # "Reset to 5V"
      n31 = call <vilib>:"Write.vi"("Values"=dbl[] [5.0], "AO Ref In"=w186) -> ("AO Ref Out"=w185:T24)  [unwired: 7 in, 1 out]
    }
    frame #2 {
      # "Wait"
      n32 = Wait (ms)(milliseconds to wait=u32 500) -> ()  [unwired: 1 out]
    }
    frame #3 {
      w202 = 7000  # Calibration_Length
      # "Sensor Ref"
      # "Reset to 0V"
      n33 = property class="App"() -> ("Disp.AllMonitors"=w211:T38)  [unwired: 2 in, 2 out]
      n34 = property class="VI"() -> ("FP.Monitor"=w210:u16)  [unwired: 2 in, 2 out]
      n35 = Unbundle By Name(w197) -> ("Tachometer"=w199:T34, "Force Sensor"=w198:T34)
      n36 = Decrement(x=w210) -> (x-1=w209:u16)
      n37 = Index Array(array=w211, index=w209) -> (element=w208:T39)
      n38 = call "Tacho_and_Force_Calibration.vi"("Force Ref In"=w198, "Tacho Ref In"=w199, "Calibration_Length"=w202) -> ("Force_calib_value"=w200:dbl, "Velocity_calib_value"=w201:dbl)  [unwired: 7 in]
      n39 = Unbundle By Name(w208) -> ("Bounds"=w207:T40)
      n40 = call <vilib>:"Write.vi"("Values"=dbl[] [0.0], "AO Ref In"=w213) -> ("AO Ref Out"=w212:T24)  [unwired: 7 in, 1 out]
      n41 = property class="VI"("Front Panel.PanelBounds"=w207) -> ()  [unwired: 2 in, 2 out]
    }
    frame #4 {
      w218 = T41 {"Task Type"=enum."HapticBump", "Phase Trial Count"=0, "Left Hand"=FALSE}  # Assessment Info
      w247 = i16 0  # Trial Nr
      w248 = Main_States."Hand choice"  # Machine State
      w232 = 0  # Loop Count
      # "Main Execution Loop"
      n42 = call "Tick Count2"() -> ("Tick Count(mSec)"=w220:u32)
      n43 = node-c288(120 ("Priority"), 1 ("Processor")) -> (w240:T12)  [unwired: 2 in]
      n44 = node-c288(i64 1000 ("Period"), 100 ("Priority"), 1 ("Processor")) -> (w246:T12)  [unwired: 1 in]
      n45 = timed-sequence {
        timing: w240 -> [_]
        timing-out: [_] -> w239
        tunnel: w243 -> [w453]
        tunnel: [w452] -> w233
        tunnel: w227 -> [w451]
        n46 = timed-flat-sequence {
          tunnel: w453 -> [w456]
          tunnel: [w455] -> w452
          tunnel: w451 -> [w454]
          n47 = node-c288() -> ()  [unwired: 1 in, 1 out]
          n48 = while {
            tunnel: w456 -> [w467]
            tunnel: [w460] -> w455
            tunnel: w454 -> [w459]
            stop <- w462 stop-if-true
            # "TCP Listener"
            # "TCP Listener"
            # "TCP \nConnection"
            # "TCP Listener Loop\nAccepts new connection\nwhenever the previous\nconnection was terminated\nuntil stop signal is set."
            # "Accept Incoming\nConnection\n(with timeout)"
            n49 = TCP Wait On Listener ("TCP Accept")(9:1000, 11:w467) -> (0:w465:errorcluster, 2:w461:string, 3:w460:refnum<k5>, 4:w466:refnum<k5>)  [unwired: 2 in, 1 out]
            n50 = case shown="No Error" w465 {
              selector: w465 -> [w477 w669]
              tunnel: w466 -> [w475 _]
              tunnel: [w478 w669] -> w463
              tunnel: w461 -> [w473 _]
              tunnel: w459 -> [w472 _]
              frame No Error {
                n51 = flat-sequence {
                  tunnel: w477 -> [w479]
                  tunnel: [w479] -> w476
                  tunnel: w475 -> [w481]
                  tunnel: [w481] -> w474
                  tunnel: w473 -> [w480]
                  frame #0 {
                    n52 = String To IP(1:w480) -> (0:w483:u32)
                    n53 = local write "TCP Error"(w479) -> ()
                    n54 = local write "Connected"(TRUE) -> ()
                    n55 = local write "Remote IP"(w483) -> ()
                  }
                }
                n56 = while {
                  tunnel: w476 -> [w504]
                  tunnel: w474 -> [w503]
                  tunnel: [w489] -> w478
                  tunnel: w472 -> [w484]
                  stop <- w496 stop-if-true
                  w490 = T42."Buffered"  # TCP Mode
                  w510 = 3  # Msg Header Length
                  # "Connection ID"
                  # "Clears Timeout \nError to avoid \nloop abortion"
                  # "TCP Message Processing Loop\nThis loops receives and processes messages\nover tcp until the stop signal is set or the\nconnection is lost.\n\nWhen the connection is lost, the loop exits\nand the outer listener loop will wait for a new\nconnection to be established."
                  # "Parse payload differently and perform different actions based on message type"
                  # "Parse header"
                  # "Receive message \npayload (timeout 1s)"
                  # "Receive header\n(timeout 1s)"
                  n57 = TCP Read(connection ID=w503, bytes to read=w510, error in (no error)=w504, 7:w490, 9:1000) -> (connection ID out=w498:refnum<k5>, data out=w512:string, error out=w509:errorcluster)
                  n58 = Unflatten From String(type=T16 {"MsgType [0]"=0, "MsgLen [1:2]"=0} ("Msg Header \nFormat"), binary string=w512, data includes array or string size? (T)=FALSE, error in (no error)=w509) -> (value=w508:T16, error out=w502:errorcluster)  [unwired: 1 in, 1 out]
                  n59 = Unbundle By Name(w508) -> ("MsgType [0]"=w506:u8, "MsgLen [1:2]"=w494:u16)
                  n60 = To Long Integer(number=w494) -> (32bit integer=w501:i32)
                  n61 = Type Cast(type=T15."Command", x=w506) -> (*(type *) &x=w500:T15)
                  n62 = TCP Read(connection ID=w498, bytes to read=w501, error in (no error)=w502, 7:w490, 9:1000) -> (connection ID out=w486:refnum<k5>, data out=w499:string, error out=w492:errorcluster)
                  n63 = case shown="\"Command\"" w500 {
                    tunnel: w492 -> [w527 w533 w549 w600 w646 w665]
                    tunnel: w499 -> [_ _ w550 w601 _ _]
                    tunnel: [FALSE ("Close") FALSE ("Close") FALSE w599 FALSE ("Close") FALSE ("Close")] -> w497
                    tunnel: [w527 w532 w541 w597 w648 w667] -> w487
                    tunnel: w486 -> [w526 w530 w540 w598 w645 w663]
                    tunnel: [w526 w529 w540 w598 w645 w662] -> w485
                    tunnel: w484 -> [_ _ w538 _ _ _]
                    frame "Invalid" {
                    }
                    frame Default {
                      # "In case of an unknown message type,\nsend '?' as reply, so the frontend can detect the version incompatibility and display an error."
                      # "Send\nReply"
                      n64 = TCP Write(connection ID=w530, data in="?", error in (no error)=w533, 9:-1 ("timeout ms (25000)")) -> (connection ID out=w529:refnum<k5>, error out=w532:errorcluster)  [unwired: 1 out]
                    }
                    frame "PatientSelect" {
                      n65 = Unflatten From String(type=T17 {"LeftHand"=FALSE, "AssessmentMode"=0, "SubjectNr"="", "DateTime"="", "PhaseTrialCount"=0, "StudyName"=""}, binary string=w550, data includes array or string size? (T)=FALSE, error in (no error)=w549) -> (value=w547:T17, error out=w542:errorcluster)  [unwired: 1 in, 1 out]
                      n66 = Unbundle By Name(w547) -> ("LeftHand"=w546:bool, "AssessmentMode"=w545:u8, "SubjectNr"=w544:string, "DateTime"=w543:string, "PhaseTrialCount"=w539:i32, "StudyName"=w536:string)
                      n67 = case shown="No Error" w542 {
                        selector: w542 -> [w563 w586]
                        tunnel: w546 -> [w567 _]
                        tunnel: w545 -> [w566 _]
                        tunnel: w544 -> [w564 _]
                        tunnel: w543 -> [w565 _]
                        tunnel: [w562 w586] -> w541
                        tunnel: w540 -> [w559 _]
                        tunnel: w539 -> [w558 _]
                        tunnel: w538 -> [w554 _]
                        tunnel: w536 -> [w552 _]
                        frame No Error {
                          # "Send\nReply"
                          n68 = flat-sequence {
                            tunnel: w567 -> [w575]
                            tunnel: w566 -> [w574]
                            tunnel: w565 -> [w572]
                            tunnel: w564 -> [w573]
                            tunnel: w563 -> [w578]
                            tunnel: w558 -> [w568]
                            tunnel: [w578] -> w557
                            tunnel: [w577] -> w556
                            tunnel: [w571] -> w555
                            tunnel: w552 -> [w570]
                            tunnel: [w581] -> w561
                            tunnel: w557 -> [w582]
                            tunnel: w556 -> [w583]
                            tunnel: w555 -> [w585]
                            tunnel: w554 -> [w584]
                            frame #0 {
                              n69 = To Word Integer(number=w568) -> (16bit integer=→"Phase Trial Count":i16)
                              n70 = Bundle By Name(cluster=T6 {"Left"=FALSE, "Mode"=enum."RangeOfMotion", "Name"="", "Timestamp"="", "StudyName"=""}, "Left"=w575, "Mode"=w574, "Name"=w573, "Timestamp"=w572, "StudyName"=w570) -> (w571:T6)
                              n71 = Select(t=Hand."Left" ("Enum"), s=w575, f=Hand."Right" ("Enum")) -> (s? t:f=w577:T2)
                              "TaskType" <- w574
                              "SubjectNr" <- w573
                              "DateTime" <- w572
                            }
                            frame #1 {
                              # "Set only after\nother vars\nwritten as it \ntriggers \nassessment\nstart"
                              n72 = Send Notification "NotifyLog"(notification=w585, notifier=w584, error in (no error)=w582) -> (error out=w581:errorcluster)  [unwired: 1 out]
                              "SelectedHand" <- w583
                            }
                          }
                          n73 = TCP Write(connection ID=w559, data in="X", error in (no error)=w561, 9:-1 ("timeout ms (25000)")) -> (error out=w562:errorcluster)  [unwired: 2 out]
                        }
                        frame Error {
                        }
                      }
                    }
                    frame "Command" {
                      n74 = Unflatten From String(type=T18 {"EmergencyStop"=FALSE, "Start"=FALSE, "Restart"=FALSE, "FrontendStarted"=FALSE, "Close"=FALSE, "StartingPosition"=0.0, "TargetPosition"=0.0, "HapticBumpForce"=0.0}, binary string=w601, data includes array or string size? (T)=FALSE, error in (no error)=w600) -> (value=w602:T18, error out=w594:errorcluster)  [unwired: 1 in, 1 out]
                      n75 = Unbundle By Name(w602) -> ("FrontendStarted"=w596:bool, "TargetPosition"=w595:sgl, "StartingPosition"=w593:sgl, "HapticBumpForce"=w587:dbl, "Start"=w591:bool, "EmergencyStop"=w590:bool, "Restart"=w589:bool, "Close"=w588:bool)
                      n76 = case shown="No Error" w594 {
                        selector: w594 -> [w612 w644]
                        tunnel: [w613 FALSE ("Close")] -> w599
                        tunnel: w588 -> [w614 _]
                        tunnel: w596 -> [w618 _]
                        tunnel: w591 -> [w617 _]
                        tunnel: w590 -> [w616 _]
                        tunnel: w589 -> [w615 _]
                        tunnel: w598 -> [w609 _]
                        tunnel: [w607 w644] -> w597
                        tunnel: w595 -> [w606 _]
                        tunnel: w593 -> [w605 _]
                        tunnel: w587 -> [w604 _]
                        frame No Error {
                          # "Send\nReply"
                          n77 = flat-sequence {
                            tunnel: w618 -> [w625]
                            tunnel: w617 -> [w622]
                            tunnel: w616 -> [w624]
                            tunnel: w615 -> [w627]
                            tunnel: [w629] -> w613
                            tunnel: w614 -> [w629]
                            tunnel: [w628] -> w608
                            tunnel: w612 -> [w628]
                            tunnel: w606 -> [w621]
                            tunnel: w605 -> [w620]
                            tunnel: w604 -> [w619]
                            frame #0 {
                              # "Only send reply for restart and stop once tdms is closed (and state machine fully reset for restart)"
                              n78 = flat-sequence {
                                tunnel: w621 -> [w634]
                                tunnel: w620 -> [w633]
                                tunnel: w619 -> [w630]
                                tunnel: w622 -> [w636]
                                frame #0 {
                                n79 = To Double Precision Float(number=w634) -> (double precision float=→"Target Position Frontend [deg]":dbl)
                                n80 = To Double Precision Float(number=w633) -> (double precision float=→"Starting Position Frontend [deg]":dbl)
                                n81 = To Double Precision Float(number=w630) -> (double precision float=→"Haptic Bump Force Frontend [N]":dbl)
                                }
                                frame #1 {
                                "StartSignal" <- w636
                                }
                              }
                              n82 = flat-sequence {
                                tunnel: w624 -> [w637]
                                tunnel: [w637] -> w623
                                frame #0 {
                                "StopSignal" <- w637
                                }
                              }
                              n83 = flat-sequence {
                                tunnel: w627 -> [w640]
                                tunnel: [w640] -> w626
                                frame #0 {
                                "RestartSignal" <- w640
                                }
                              }
                              n84 = case shown="True" w626 {
                                frame False {
                                }
                                frame True {
                                n85 = while {
                                stop <- w641 continue-if-true
                                n86 = local read "RestartSignal"() -> (w641:bool)
                                n87 = Wait (ms)(milliseconds to wait=u32 30) -> ()  [unwired: 1 out]
                                }
                                }
                              }
                              n88 = case shown="True" w623 {
                                frame False {
                                }
                                frame True {
                                n89 = while {
                                stop <- w638 continue-if-true
                                n90 = local read "LogFileOpen"() -> (w638:bool)
                                n91 = Wait (ms)(milliseconds to wait=u32 30) -> ()  [unwired: 1 out]
                                }
                                }
                              }
                              "FrontendStartedSignal" <- w625
                            }
                          }
                          n92 = TCP Write(connection ID=w609, data in="X", error in (no error)=w608, 9:-1 ("timeout ms (25000)")) -> (error out=w607:errorcluster)  [unwired: 2 out]
                        }
                        frame Error {
                        }
                      }
                    }
                    frame "Skip" {
                      # "Send\nReply"
                      n93 = flat-sequence {
                        tunnel: [w652] -> w647
                        tunnel: w646 -> [w652]
                        frame #0 {
                          "SkipSignal" <- TRUE ("SkipSignal")
                        }
                      }
                      n94 = TCP Write(connection ID=w645, data in="X", error in (no error)=w647, 9:-1 ("timeout ms (25000)")) -> (error out=w648:errorcluster)  [unwired: 2 out]
                    }
                    frame "BackendInfoReq" {
                      # "Send\nReply"
                      n95 = local read "Largest USB Partition Path"() -> (w655:path)
                      n96 = Path To String(path=w655) -> (string=w654:string)
                      n97 = Bundle By Name(cluster=T19 {"ProtocolVersion"=2, "DataPath"=""} ("Cluster"), "ProtocolVersion"=u16 2, "DataPath"=w654) -> (w657:T19)
                      n98 = Flatten To String(anything=w657, error in (no error)=w665) -> (data string=w659:string, error out=w664:errorcluster)  [unwired: 2 in, 1 out]
                      n99 = Concatenate Strings("Y" ("string"), w659) -> (w660:string)
                      n100 = TCP Write(connection ID=w663, data in=w660, error in (no error)=w664, 9:-1 ("timeout ms (25000)")) -> (connection ID out=w662:refnum<k5>, error out=w667:errorcluster)  [unwired: 1 out]
                    }
                  }
                  n101 = call <vilib>:"Clear Errors.vi"("error in (no error)"=w487, "specific error code to clear (0: all)"=56) -> ("error out"=w488:errorcluster)  [unwired: 4 in, 1 out]
                  n102 = flat-sequence "Stop Signal" {
                    tunnel: [w518] -> w493
                    tunnel: w488 -> [w518]
                    tunnel: w497 -> [w521]
                    tunnel: [w522] -> w496
                    frame #0 {
                      # "Reset connection\non error"
                      n103 = local read "StopRequested"() -> (w523:bool)
                      n104 = case shown="No Error" w518 {
                        tunnel: [FALSE TRUE] -> w519
                        frame No Error {
                        }
                        frame Error {
                        }
                      }
                      n105 = Or(x=w519, y=w521) -> (x .or. y?=w520:bool)
                      n106 = Or(x=w520, y=w523) -> (x .or. y?=w522:bool)
                    }
                  }
                  n107 = case shown="True" w496 {
                    tunnel: w485 -> [_ w517]
                    tunnel: w493 -> [w514 w516]
                    tunnel: [w514 w515] -> w489
                    frame False {
                    }
                    frame True {
                      n108 = TCP Close Connection "TCP Close"(connection ID=w517, error in (no error)=w516) -> (error out=w515:errorcluster)  [unwired: 1 in, 1 out]
                    }
                  }
                  "Error which lead\nto TCP close" <- w489
                }
              }
              frame Error {
                # "Probably timed out,\nbecause nobody connected\n-> try again in next iteration"
              }
            }
            n109 = flat-sequence "Stop Signal" {
              tunnel: [w471] -> w462
              tunnel: w463 -> [w469]
              frame #0 {
                n110 = local read "StopRequested"() -> (w471:bool)
                n111 = local write "Connected"(FALSE) -> ()
                n112 = local write "Remote IP"(u32 0 ("Remote IP")) -> ()
                "TCP Error" <- w469
              }
            }
          }
          n113 = node-c288() -> ()  [unwired: 1 in, 1 out]
        }
      }
      n114 = timed-loop {
        timing: w246 -> [_]
        timing-out: [_] -> w245
        tunnel: w244 -> [w683]
        tunnel: [w682] -> w234
        stop <- w680 stop-if-true
        # "UDP Socket"
        # "UDP Sending Loop"
        n115 = node-c288() -> ()  [unwired: 1 in, 1 out]
        n116 = call "UdpDataGlobal.vi"("Action"=UdpGlobalActions."Read") -> ("UDP Robot State"=w676:T43)  [unwired: 26 in]
        n117 = local read "Remote IP"() -> (w679:u32)
        n118 = Flatten To String(anything=w676, prepend array or string size? (T)=FALSE) -> (data string=w686:string, error out=w685:errorcluster)  [unwired: 2 in, 1 out]
        n119 = UDP Write(address=w679, port or service name="UDP Destination Port", connection ID=w683, data in=w686, 8:w685, 9:5 ("specific error code to clear (0: all)")) -> (error out=w684:errorcluster, 3:w682:refnum<k16>)
        n120 = flat-sequence "Stop Signal" {
          tunnel: w684 -> [w688]
          tunnel: [w689] -> w680
          tunnel: [w688] -> w678
          frame #0 {
            n121 = local read "StopRequested"() -> (w689:bool)
          }
        }
        n122 = node-c288() -> ()  [unwired: 1 in, 1 out]
        "UDP Error" <- w678
      }
      n123 = node-c288(i64 1000 ("Period"), 1000 ("Priority"), 0 ("Processor")) -> (w253:T12)  [unwired: 1 in]
      n124 = timed-loop "Main Control Loop" {
        timing: w253 -> [_]
        timing-out: [_] -> w252
        tunnel: [w742] -> w226
        shift-right: [w729] -> _
        shift-left: w248 -> [w726]
        shift-right: [w727] -> _
        shift-left: w232 -> [w728]
        shift-right: [w735] -> _
        shift-left: w247 -> [w731]
        tunnel: w222 -> [w725]
        tunnel: w221 -> [w724]
        tunnel: w220 -> [w723]
        tunnel: w219 -> [w716]
        shift-right: [w707] -> _
        shift-left: w218 -> [w712]
        tunnel: w217 -> [w705]
        tunnel: w216 -> [w704]
        shift-right: [w702] -> _
        shift-left: 0.0 -> [w701]
        stop <- w739 stop-if-true
        # "Task Info"
        # "Machine State"
        # "Trial Nr"
        # "Loop Count"
        n125 = node-c288() -> (w738:bool, w743:i64)  [unwired: 1 in, 14 out]
        n126 = flat-sequence {
          tunnel: w743 -> [w757]
          tunnel: [w754] -> w722
          tunnel: w726 -> [w754]
          tunnel: w738 -> [w765]
          tunnel: [w763] -> w720
          tunnel: w728 -> [w763]
          tunnel: [w753] -> w718
          tunnel: w731 -> [w753]
          tunnel: w725 -> [w746]
          tunnel: w724 -> [w747]
          tunnel: w723 -> [w752]
          tunnel: [w749] -> w715
          tunnel: w712 -> [w748]
          tunnel: [w748] -> w711
          tunnel: w704 -> [w745]
          tunnel: w701 -> [w744]
          tunnel: [w744] -> w700
          tunnel: w722 -> [w806]
          tunnel: [w806] -> w721
          tunnel: w720 -> [w805]
          tunnel: [w805] -> w719
          tunnel: w718 -> [w778]
          tunnel: [w778] -> w717
          tunnel: w716 -> [w787]
          tunnel: w715 -> [w769]
          tunnel: [w769] -> w714
          tunnel: w711 -> [w768]
          tunnel: [w768] -> w710
          tunnel: w700 -> [w766]
          tunnel: [w766] -> w698
          tunnel: w721 -> [w813]
          tunnel: [w813] -> w734
          tunnel: w719 -> [w814]
          tunnel: [w814] -> w733
          tunnel: [w812] -> w732
          tunnel: w717 -> [w811]
          tunnel: [w811] -> w730
          tunnel: w714 -> [w810]
          tunnel: [w810] -> w713
          tunnel: w710 -> [w809]
          tunnel: [w808] -> w709
          tunnel: [w807] -> w699
          tunnel: w698 -> [w807]
          tunnel: [w850] -> w741
          tunnel: w734 -> [w848]
          tunnel: [w844] -> w740
          tunnel: w733 -> [w845]
          tunnel: [w843] -> w737
          tunnel: [w849] -> w736
          tunnel: w732 -> [w847]
          tunnel: w730 -> [w846]
          tunnel: w713 -> [w841]
          tunnel: w709 -> [w842]
          tunnel: [w842] -> w708
          tunnel: [w841] -> w706
          tunnel: [w840] -> w703
          tunnel: w699 -> [w839]
          tunnel: w741 -> [w1499]
          tunnel: w740 -> [w1492]
          tunnel: w737 -> [w1506]
          tunnel: w736 -> [w1501]
          tunnel: [w1507] -> w742
          tunnel: [w1495] -> w729
          tunnel: [w1504] -> w739
          tunnel: [w1506] -> w727
          tunnel: [w1501] -> w735
          tunnel: w708 -> [w1493]
          tunnel: [w1493] -> w707
          tunnel: w706 -> [w1491]
          tunnel: w705 -> [w1490]
          tunnel: w703 -> [w1488]
          tunnel: [w1488] -> w702
          frame #0 {
            # "Time since first main loop iteration (s)"
            # "Period (s)"
            # "Calculate position/velocity etc"
            n127 = To Double Precision Float(number=w757) -> (double precision float=w758:dbl)
            n128 = To Double Precision Float(number=1000000) -> (double precision float=w756:dbl)
            n129 = call "Tick Count"() -> ("Tick Count(mSec)"=w764:u32)
            n130 = Divide(x=w758, y=w756) -> (x/y=w751:dbl)
            n131 = Subtract(x=w764, y=w752) -> (x-y=w760:u32)
            n132 = To Double Precision Float(number=w760) -> (double precision float=w762:dbl)
            n133 = To Double Precision Float(number=u32 1000 ("y")) -> (double precision float=w761:dbl)
            n134 = Divide(x=w762, y=w761) -> (x/y=w750:dbl)
            n135 = call "ReadAndPreprocessSensorValues.vi"("Sensor References"=w747, "Force_calib_value"=w746, "Velocity_calib_value"=w745, "Control Loop Period [s]"=w751, "Time [s]"=w750) -> ("RobotStateType"=w749:T1)  [unwired: 6 in]
            "RobotState" <- w749
            "Finished late?" <- w765
          }
          frame #1 {
            # "Display target array on front panel"
            # "Robot State"
            # "Write state To cluster that will be published over UDP"
            # "Writing state to Log Queue (rt fifo) for TDMS logging"
            # "Machine State"
            # "Task Info"
            # "Trial Nr"
            # "Loop Count"
            # "Store current state for logging"
            n136 = Unbundle By Name(w769) -> ("Time [s]"=w770:dbl, "Position [deg]"=w771:dbl)
            n137 = local read "Target Position [deg]"() -> (w786:dbl)
            n138 = local read "Target state?"() -> (w798:bool)
            n139 = local read "FrontendStartedSignal"() -> (w791:bool)
            n140 = Unbundle By Name(w769) -> ("Velocity [deg/s]"=w773:dbl, "Current [A]"=w772:dbl)
            n141 = local read "Starting position"() -> (w796:dbl)
            n142 = Unbundle By Name(w769) -> ("Voltage force"=w774:dbl, "Force"=w775:dbl, "Force filtered"=w776:dbl, "Velocity unfiltered [deg/s]"=w777:dbl)
            n143 = Unbundle By Name(w769) -> ("Position [deg]"=w785:dbl, "Force filtered"=w781:dbl, "Time [s]"=w784:dbl)
            n144 = local read "Starting position"() -> (w779:dbl)
            n145 = local read "Target Position [deg]"() -> (w780:dbl)
            n146 = local read "Target state?"() -> (w782:bool)
            n147 = local read "ROM State"() -> (w783:T3)
            n148 = local read "LogFileOpen"() -> (w802:bool)
            n149 = local read "TaskFinished"() -> (w800:bool)
            n150 = local read "Target Array"() -> (→"Target Array":dbl[])
            n151 = Not(x=w802) -> (.not. x?=w801:bool)
            n152 = Boolean To (0,1)(Boolean=w798) -> (0, 1=w789:i16)
            n153 = Boolean To (0,1)(Boolean=w791) -> (0, 1=w795:i16)
            n154 = And(x=w800, y=w801) -> (x .and. y?=w803:bool)
            n155 = To Double Precision Float(number=w789) -> (double precision float=w790:dbl)
            n156 = To Double Precision Float(number=w795) -> (double precision float=w792:dbl)
            n157 = local read "Flexion"() -> (w797:bool)
            n158 = local read "ROM State"() -> (w799:T3)
            n159 = call "UdpDataGlobal.vi"("Position"=w785, "Starting Position"=w779, "Target Position"=w780, "Force"=w781, "TargetState"=w782, "RomState"=w783, "Time"=w784, "Finished"=w803, "Flexion"=w797, "Trial Nr"=w778, "Action"=UdpGlobalActions."Write") -> ()  [unwired: 16 in, 1 out]
            n160 = To Double Precision Float(number=w778) -> (double precision float=w793:dbl)
            n161 = To Double Precision Float(number=w799) -> (double precision float=w794:dbl)
            n162 = Build Array(w770, w771, w786, w790, w792, w793, w773, w772, w796, w774, w775, w776, w777, w794) -> (w788:dbl[])
            n163 = RT FIFO Write(0:w787, 1:w788) -> ()  [unwired: 3 in, 4 out]
          }
          frame #2 {
            # "Initialize Task Info and Start Task"
            n164 = case "Initialize Task Info from FrontEnd before Task begins" shown="\"Hand choice\"" w813 {
              tunnel: [TRUE w819] -> w812
              tunnel: w809 -> [w815 w818]
              tunnel: [w815 w817] -> w808
              frame Default {
              }
              frame "Hand choice" {
                n165 = local read "SelectedHand"() -> (w820:T2)
                n166 = case shown="Default" w820 {
                  selector: w820 -> [_ w835]
                  tunnel: [FALSE TRUE] -> w819
                  tunnel: w818 -> [w821 _]
                  tunnel: [w821 w826] -> w817
                  frame "None" {
                  }
                  frame Default {
                    w827 = T41 {"Task Type"=enum."HapticBump", "Phase Trial Count"=0, "Left Hand"=FALSE}  # Task Info
                    n167 = local read "Phase Trial Count"() -> (w831:i16)
                    n168 = local read "TaskType"() -> (w828:T5)
                    n169 = local write "ROM State"(ROM_States."Active" ("Enum")) -> ()
                    n170 = local write "Starting Position Frontend [deg]"(0.0 ("Target Position Frontend [deg]")) -> ()
                    n171 = local write "Target Position Frontend [deg]"(0.0 ("Target Position Frontend [deg]")) -> ()
                    n172 = local write "Haptic Bump Force Frontend [N]"(0.0) -> ()
                    n173 = case shown="\"PositionMatching\"" w828 {
                      tunnel: [i16 1 i16 2] -> w832
                      frame Default {
                      }
                      frame "PositionMatching" {
                      }
                    }
                    n174 = Equal?(x=w835, y=Hand."Left" ("Enum")) -> (x = y?=w830:bool)
                    "LeftHand" <- w830
                    n175 = Max & Min(x=w832, y=w831) -> (max(x,y)=w829:i16)  [unwired: 1 out]
                    n176 = Bundle By Name(cluster=w827, "Task Type"=w828, "Phase Trial Count"=w829, "Left Hand"=w830) -> (w826:T41)
                  }
                }
              }
            }
          }
          frame #3 {
            # "Robot State"
            # "Task Info"
            # "Machine State"
            # "StartTask"
            # "Loop Count"
            # "Trial Nr"
            # "State Machine"
            n177 = case shown="\"Show target\"" w848 {
              selector: w848 -> [w858 _ w893 _ _ w1475]
              tunnel: [w857 Main_States."StartTrial" ("Task states") w903 w1125 Main_States."WaitingForRestart" ("Task states") w1474] -> w850
              tunnel: [0.0 ("u") 0.0 w906 w1135 0.0 ("u") 0.0 ("u")] -> w844
              tunnel: w845 -> [_ _ _ w1133 _ _]
              tunnel: [w853 w865 0 w1132 0 0] -> w843
              tunnel: [w854 w860 w902 w1137 w1468 w1480] -> w849
              tunnel: w846 -> [_ _ w894 w1138 w1468 w1480]
              tunnel: w847 -> [w852 _ _ _ _ _]
              tunnel: w841 -> [_ _ w901 w1126 _ _]
              tunnel: w842 -> [_ w863 w895 w1127 _ _]
              tunnel: [w851 w859 w892 w1122 w1463 w1473] -> w840
              tunnel: w839 -> [w851 w859 w892 w1121 w1463 w1473]
              frame "Hand choice", Default {
                w853 = 0  # Loop Count
                w854 = i16 1  # Trial Nr
                n178 = Select(t=Main_States."StartTask" ("Task states"), s=w852, f=w858) -> (s? t:f=w857:T4)
              }
              frame "StartTask" {
                w860 = i16 1  # Trial Nr
                w865 = 0  # Loop Count
                n179 = Unbundle By Name(w863) -> ("Task Type"=w864:T5)
                n180 = case "Precalculating Target Arrays" shown="\"PositionMatching\"" w864 {
                  tunnel: w863 -> [_ w873 w881 w891]
                  frame Default {
                  }
                  frame "Motor" {
                    w869 = dbl[] [30.0, 70.0]
                    n181 = Unbundle By Name(w873) -> ("Left Hand"=w868:bool, "Phase Trial Count"=w872:i16)
                    n182 = To Long Integer(number=w872) -> (32bit integer=w867:i32)
                    n183 = Negate(x=w869) -> (-x=w870:dbl[])
                    n184 = Select(t=w869, s=w868, f=w870) -> (s? t:f=w871:dbl[])
                    n185 = call "RandomizeTargetSequence.vi"("NumRepetitions"=w867, "Inputs"=w871) -> ("Target Array"=w866:dbl[])  [unwired: 9 in]
                    n186 = local write "Target Array"(w866) -> ()
                  }
                  frame "PreciseReaching" {
                    w876 = dbl[] [50.0, 70.0]
                    n187 = Unbundle By Name(w881) -> ("Left Hand"=w875:bool, "Phase Trial Count"=w880:i16)
                    n188 = To Long Integer(number=w880) -> (32bit integer=w874:i32)
                    n189 = Negate(x=w876) -> (-x=w877:dbl[])
                    n190 = Select(t=w876, s=w875, f=w877) -> (s? t:f=w878:dbl[])
                    n191 = call "RandomizeTargetSequence.vi"("NumRepetitions"=w874, "Inputs"=w878) -> ("Target Array"=w879:dbl[])  [unwired: 9 in]
                    n192 = local write "Target Array"(w879) -> ()
                  }
                  frame "PositionMatching" {
                    w884 = 30.0
                    w888 = 30.0  # Max Range
                    w889 = 10.0  # Min Range
                    # "Precompute starting position here,\nas target array depends on starting position"
                    n193 = Unbundle By Name(w891) -> ("Left Hand"=w883:bool, "Phase Trial Count"=w890:i16)
                    n194 = Negate(x=w884) -> (-x=w885:dbl)
                    n195 = Select(t=w884, s=w883, f=w885) -> (s? t:f=w882:dbl)
                    n196 = To Long Integer(number=w890) -> (32bit integer=w886:i32)
                    n197 = call "GenerateTargetArrayFromInterval.vi"("Max Range"=w888, "Min Range"=w889, "Left Hand"=w883, "Num Steps (Inclusive)"=w886, "Starting Position"=w882) -> ("Target Array"=w887:dbl[])
                    n198 = local write "Starting position"(w882) -> ()
                    n199 = local write "Target Array"(w887) -> ()
                  }
                }
              }
              frame "StartTrial" {
                # "Phase Trial Count"
                # "Trial Nr [IN]"
                # "Starting Position"
                n200 = local read "StartSignal"() -> (w899:bool)
                n201 = Unbundle By Name(w895) -> ("Task Type"=w900:T5)
                n202 = First Call?() -> (First Call?: T/F=w898:bool)
                n203 = call <vilib>:"Boolean Crossing PtByPt.vi"("initialize"=w898, "direction"=enum16{"either", "false-true", "true-false"}."false-true", "input"=w899) -> ("crossing"=w897:bool)
                n204 = case "Calculating starting Position and Target Arrays" shown="\"PassiveMatching\"..\"TeachAndReproduce\"" w900 {
                  tunnel: [w1046 0.0 ("f") w1084 w1100 w1110 w1111 w1114 w1120] -> w905
                  tunnel: w894 -> [_ w1073 w1087 w1103 _ _ _ w1118]
                  tunnel: w895 -> [w1045 w1072 w1083 w1098 w1107 _ _ _]
                  frame "RangeOfMotion" {
                    n205 = local read "ROM State"() -> (w1047:T3)
                    n206 = case shown="\"AutomaticPassive\"" w1047 {
                      tunnel: [w1051 w1068] -> w1046
                      tunnel: w1045 -> [w1049 w1067]
                      frame "AutomaticPassive" {
                        # "Determine middle between max and\nmin range to start sinewave from"
                        # "If limit is above 82 the arm can crash\ninto the end of the guidance if the \npatient has a big range of motion"
                        n207 = Unbundle By Name(w1049) -> ("Left Hand"=w1048:bool)
                        n208 = local read "ROM max"() -> (w1053:dbl)
                        n209 = call "angle_limit.vi"() -> ("LimitAngle"=w1050:dbl)  [unwired: 2 in]
                        n210 = case "Limit max Angle" shown="False" w1048 {
                          tunnel: w1053 -> [w1057 w1064]
                          tunnel: [w1060 w1063] -> w1052
                          tunnel: w1050 -> [w1059 w1062]
                          frame False {
                            n211 = Negate(x=w1059) -> (-x=w1058:dbl)
                            n212 = Greater?(x=w1057, y=w1058) -> (0:w1061:bool)
                            n213 = Select(t=w1057, s=w1061, f=w1058) -> (s? t:f=w1060:dbl)
                          }
                          frame True {
                            n214 = Less?(x=w1064, y=w1062) -> (x < y?=w1065:bool)
                            n215 = Select(t=w1064, s=w1065, f=w1062) -> (s? t:f=w1063:dbl)
                          }
                        }
                        n216 = local write "ROM max"(w1052) -> ()
                        n217 = local read "ROM min"() -> (w1054:dbl)
                        n218 = Add(x=w1052, y=w1054) -> (x+y=w1055:dbl)
                        n219 = Divide(x=w1055, y=2.0) -> (x/y=w1051:dbl)
                        "Zero Position" <- w1051
                        n220 = local write "Starting position"(w1051) -> ()
                      }
                      frame "Active", "Passive", Default {
                        w1070 = 30.0
                        n221 = Unbundle By Name(w1067) -> ("Left Hand"=w1066:bool)
                        n222 = Negate(x=w1070) -> (-x=w1069:dbl)
                        n223 = Select(t=w1070, s=w1066, f=w1069) -> (s? t:f=w1068:dbl)
                      }
                    }
                  }
                  frame "Force" {
                    # "Only write if the trial nr\nhas changed and at the \nfirst iteration\n(due to performace reasons)"
                    n224 = Unbundle By Name(w1072) -> ("Phase Trial Count"=w1071:i16)
                    n225 = feedback-in #1(w1073) -> ()
                    n226 = feedback #1(i16 -1 ("Trial Nr")) -> (w1074:i16)
                    n227 = Not Equal?(x=w1074, y=w1073) -> (x != y?=w1076:bool)
                    n228 = case "Set Flexion Flag" shown="True" w1076 {
                      tunnel: w1073 -> [_ w1079]
                      tunnel: w1071 -> [_ w1078]
                      frame False {
                      }
                      frame True {
                        n229 = Less Or Equal?(x=w1079, y=w1078) -> (x <= y?=→"Flexion":bool)
                      }
                    }
                  }
                  frame "Motor" {
                    # "Initialized during TaskState = StartTask"
                    # "Left Hand?"
                    # "Flexion?"
                    # "Choose the starting position based on the target position"
                    n230 = Unbundle By Name(w1083) -> ("Left Hand"=w1082:bool)
                    n231 = local read "Target Array"() -> (w1081:dbl[])
                    n232 = Decrement(x=w1087) -> (x-1=w1086:i16)
                    n233 = To Long Integer(number=w1086) -> (32bit integer=w1085:i32)
                    n234 = Index Array(array=w1081, index=w1085) -> (element=w1088:dbl)
                    n235 = local write "Target Position [deg]"(w1088) -> ()
                    n236 = Absolute Value(x=w1088) -> (abs(x)=w1094:dbl)
                    n237 = Less?(x=w1094, y=45.0) -> (x < y?=w1093:bool)
                    n238 = Select(t=70.0 ("y"), s=w1093, f=30.0 ("y")) -> (s? t:f=w1089:dbl)
                    n239 = Negate(x=w1089) -> (-x=w1090:dbl)
                    n240 = Select(t=w1089, s=w1082, f=w1090) -> (s? t:f=w1084:dbl)
                    n241 = local write "Starting position"(w1084) -> ()
                  }
                  frame "PreciseReaching" {
                    w1099 = 30.0
                    # "Initialized during TaskState = StartTask"
                    n242 = Unbundle By Name(w1098) -> ("Left Hand"=w1097:bool)
                    n243 = Negate(x=w1099) -> (-x=w1105:dbl)
                    n244 = local read "Target Array"() -> (w1096:dbl[])
                    n245 = Select(t=w1099, s=w1097, f=w1105) -> (s? t:f=w1100:dbl)
                    n246 = local write "Starting position"(w1100) -> ()
                    n247 = Decrement(x=w1103) -> (x-1=w1102:i16)
                    n248 = To Long Integer(number=w1102) -> (32bit integer=w1101:i32)
                    n249 = Index Array(array=w1096, index=w1101) -> (element=w1104:dbl)
                    n250 = local write "Target Position [deg]"(w1104) -> ()
                  }
                  frame "Sensorimotor" {
                    w1109 = 45.0
                    n251 = Unbundle By Name(w1107) -> ("Left Hand"=w1106:bool)
                    n252 = Negate(x=w1109) -> (-x=w1108:dbl)
                    n253 = Select(t=w1109, s=w1106, f=w1108) -> (s? t:f=w1110:dbl)
                    n254 = local write "Starting position"(w1110) -> ()
                    n255 = local write "Target Position [deg]"(w1110) -> ()
                  }
                  frame "PassiveMatching".."TeachAndReproduce" {
                    n256 = local read "Starting Position Frontend [deg]"() -> (w1111:dbl)
                    n257 = local read "Target Position Frontend [deg]"() -> (w1112:dbl)
                    n258 = local write "Starting position"(w1111) -> ()
                    n259 = local write "Target Position [deg]"(w1112) -> ()
                  }
                  frame "HapticBump" {
                    n260 = local read "Starting Position Frontend [deg]"() -> (w1114:dbl)
                    n261 = local read "Target Position Frontend [deg]"() -> (w1115:dbl)
                    n262 = local read "Haptic Bump Force Frontend [N]"() -> (w1113:dbl)
                    n263 = local write "Haptic Bump Force [N]"(w1113) -> ()
                    n264 = local write "Starting position"(w1114) -> ()
                    n265 = local write "Target Position [deg]"(w1115) -> ()
                  }
                  frame "PositionMatching" {
                    # "Read actual target element from array\n(array starts from 0, trial from 1)"
                    # "Defined during TaskState = StartTask"
                    n266 = local read "Target Array"() -> (w1119:dbl[])
                    n267 = Decrement(x=w1118) -> (x-1=w1117:i16)
                    n268 = local read "Starting position"() -> (w1120:dbl)
                    n269 = Index Array(array=w1119, index=w1117) -> (element=w1116:dbl)
                    n270 = local write "Target Position [deg]"(w1116) -> ()
                  }
                }
                n271 = case shown="False" w899 {
                  tunnel: [w911 w944] -> w903
                  tunnel: [0.0 ("u") w948] -> w906
                  tunnel: w897 -> [_ w947]
                  tunnel: w905 -> [_ w942]
                  tunnel: w893 -> [w912 _]
                  tunnel: w894 -> [w909 w941]
                  tunnel: [w908 w941] -> w902
                  tunnel: w901 -> [_ w940]
                  tunnel: w895 -> [w907 w939]
                  frame False {
                    n272 = local read "SkipSignal"() -> (w910:bool)
                    n273 = case shown="True" w910 {
                      tunnel: w912 -> [w915 _]
                      tunnel: [w915 w923] -> w911
                      tunnel: w909 -> [w914 w922]
                      tunnel: [w914 w919] -> w908
                      tunnel: w907 -> [_ w918]
                      frame False {
                      }
                      frame True {
                        n274 = Unbundle By Name(w918) -> ("Phase Trial Count"=w916:i16, "Task Type"=w917:T5)
                        n275 = case shown="Default" w917 {
                          tunnel: w922 -> [w927 w934]
                          tunnel: [FALSE w932] -> w921
                          tunnel: [w927 w936] -> w919
                          tunnel: w916 -> [_ w929]
                          frame Default {
                          }
                          frame "Sensorimotor" {
                            n276 = Quotient & Remainder(x=w934, y=w929) -> (x-y*floor(x/y)=w935:i16)  [unwired: 1 out]
                            n277 = Increment(x=w929) -> (x+1=w930:i16)
                            n278 = Equal? "firstTrialOfPhase?"(x=i16 1, y=w935) -> (x = y?=w933:bool)
                            n279 = Greater? "afterFirstInLastPhase?"(x=w934, y=w930) -> (0:w932:bool)
                            n280 = Or(x=w933, y=w932) -> (x .or. y?=w931:bool)
                            n281 = Select(t=w934, s=w931, f=w930) -> (s? t:f=w936:i16)
                          }
                        }
                        n282 = case shown="True" w921 {
                          tunnel: [Main_States."StartTrial" ("Task states") Main_States."Resetting" ("Task states")] -> w923
                          frame False {
                            # "Skip Phase"
                          }
                          frame True {
                            # "Skip to Finished"
                            n283 = local write "TaskFinished"(TRUE ("AssessmentFinished")) -> ()
                          }
                        }
                        n284 = local write "SkipSignal"(FALSE ("SkipSignal")) -> ()
                      }
                    }
                  }
                  frame True {
                    # "Trial Nr [OUT]"
                    # "In Position Matching & PassiveMatching\nTargetState is set later"
                    n285 = Unbundle By Name(w939) -> ("Task Type"=w938:T5)
                    n286 = case "Move to the Starting Position" shown="\"TeachAndReproduce\"" w938 {
                      tunnel: w947 -> [w953 w1008 w1031]
                      tunnel: [0.0 w1004 w1027] -> w948
                      tunnel: w942 -> [_ w1009 w1032]
                      tunnel: [w954 w1007 w1030] -> w943
                      tunnel: w940 -> [_ w999 w1022]
                      frame "Force" {
                        # "Nonblocking wait for realtime systems.\nLoop will keep running until the timer\nhas reached the set amount.\nThis wait is for the patient to prepare"
                        n287 = feedback #2(TRUE ("done")) -> (w952:bool)
                        n288 = Or(x=w953, y=w952) -> (x .or. y?=w951:bool)
                        n289 = xnode "Elapsed Timer"("reset"=w951) -> ("elapsed time (ms)"=w956:i32)  [unwired: 2 in, 1 out]
                        n290 = Greater Or Equal?(x=w956, y=3000 ("milliseconds to wait")) -> (x >= y?=w954:bool)
                        n291 = feedback-in #2(w954) -> ()
                      }
                      frame Default {
                        n292 = Unbundle By Name(w999) -> ("Position [deg]"=w998:dbl)
                        n293 = feedback #3(TRUE ("profile complete?")) -> (w1006:bool)
                        n294 = Or(x=w1008, y=w1006) -> (x .or. y?=w1012:bool)
                        n295 = feedback #4() -> (w1011:cluster{"time (s)":dbl, "setpoint":dbl}[])  [unwired: 1 in]
                        n296 = case shown="True" w1012 {
                          tunnel: [w1013 w1018] -> w1010
                          tunnel: w998 -> [_ w1015]
                          tunnel: w1011 -> [w1013 _]
                          tunnel: w1009 -> [_ w1016]
                          frame False {
                          }
                          frame True {
                            n297 = call "motion_create_minimum_jerk.vi"("Initial Position"=w1015, "Final Position"=w1016, "Initial Time [s]"=0.0, "Final Time [s]"=3.0, "Delta Time [s]"=0.01) -> ("Profile"=w1018:cluster{"time (s)":dbl, "setpoint":dbl}[])  [unwired: 10 in]
                          }
                        }
                        n298 = feedback-in #4(w1010) -> ()
                        n299 = Unbundle By Name(w999) -> ("Position [deg]"=w1000:dbl, "Velocity [deg/s]"=w1001:dbl, "Control Loop Period [s]"=w1002:dbl)
                        n300 = call <vilib>:"PID Setpoint Profile.vi"("reinitialize? (F)"=w1012, "setpoint profile"=w1010) -> ("profile complete?"=w1007:bool, "setpoint"=w1003:dbl)  [unwired: 4 in, 2 out]
                        n301 = feedback-in #3(w1007) -> ()
                        n302 = call "min_jerk_params.vi"() -> ("PID Settings"=w997:T44)  [unwired: 19 in]
                        n303 = call "ENPID.vi"("PID Settings"=w997, "r"=w1003, "y"=w1000, "dy/dt"=w1001, "dt (s)"=w1002) -> ("u"=w1004:dbl)  [unwired: 13 in, 1 out]
                      }
                      frame "TeachAndReproduce" {
                        n304 = Unbundle By Name(w1022) -> ("Position [deg]"=w1021:dbl)
                        n305 = feedback #5(TRUE ("profile complete?")) -> (w1029:bool)
                        n306 = Or(x=w1031, y=w1029) -> (x .or. y?=w1035:bool)
                        n307 = feedback #6() -> (w1034:cluster{"time (s)":dbl, "setpoint":dbl}[])  [unwired: 1 in]
                        n308 = case shown="True" w1035 {
                          tunnel: [w1036 w1043] -> w1033
                          tunnel: w1021 -> [_ w1040]
                          tunnel: w1034 -> [w1036 _]
                          tunnel: w1032 -> [_ w1041]
                          frame False {
                          }
                          frame True {
                            n309 = local read "Target Position Frontend [deg]"() -> (w1037:dbl)
                            n310 = call "min_jerk_trajectory_start_target_start.vi"("Initial Position"=w1040, "Start Position"=w1041, "Target Position"=w1037, "Initial Time [s]"=0.0, "Time For 1 Transition [s]"=3.0, "Pause duration at target [s]"=3.0, "Delta Time [s]"=0.01) -> ("Profile"=w1043:cluster{"time (s)":dbl, "setpoint":dbl}[])  [unwired: 8 in]
                          }
                        }
                        n311 = feedback-in #6(w1033) -> ()
                        n312 = Unbundle By Name(w1022) -> ("Position [deg]"=w1023:dbl, "Velocity [deg/s]"=w1024:dbl, "Control Loop Period [s]"=w1025:dbl)
                        n313 = call <vilib>:"PID Setpoint Profile.vi"("reinitialize? (F)"=w1035, "setpoint profile"=w1033) -> ("profile complete?"=w1030:bool, "setpoint"=w1026:dbl)  [unwired: 4 in, 2 out]
                        n314 = feedback-in #5(w1030) -> ()
                        n315 = call "min_jerk_params.vi"() -> ("PID Settings"=w1020:T44)  [unwired: 19 in]
                        n316 = call "ENPID.vi"("PID Settings"=w1020, "r"=w1026, "y"=w1023, "dy/dt"=w1024, "dt (s)"=w1025) -> ("u"=w1027:dbl)  [unwired: 13 in, 1 out]
                      }
                    }
                    n317 = case shown="Default" w938 {
                      tunnel: w943 -> [_ w950]
                      frame "PositionMatching", "PassiveMatching" {
                      }
                      frame Default {
                        n318 = local write "Target state?"(w950) -> ()
                      }
                    }
                    n319 = case shown="True" w943 {
                      frame False {
                      }
                      frame True {
                        w949 = FALSE
                        n320 = local write "StartSignal"(w949) -> ()
                        n321 = local write "SkipSignal"(w949) -> ()
                      }
                    }
                    n322 = Select(t=Main_States."Show target" ("Task states"), s=w943, f=Main_States."StartTrial" ("Task states")) -> (s? t:f=w944:T4)
                  }
                }
              }
              frame "Show target" {
                # "Trial Nr"
                # "Loop Count"
                # "Selects next state depending\non if a trial is finished and\nif the max amount of trials\nhas been reached"
                # "Trial Finished"
                # "Max Trial reached"
                # "Current"
                # "Current Setpoint"
                # "In range"
                # "Trial Nr"
                n323 = Unbundle By Name(w1127) -> ("Task Type"=w1128:T5)
                n324 = Unbundle By Name(w1126) -> ("Position [deg]"=w1129:dbl)
                n325 = disable-structure shown="Enabled" {
                  disable-tunnel: [w1460 0.0 ("Current")] -> w1124
                  disable-tunnel: w1129 -> [w1459 _]
                  frame Enabled {
                    # "Position"
                    # "Disable this Subdiagram to deactivate gravity compensation"
                    n326 = call "GravityCompensation.vi"("Position [deg]"=w1459) -> ("Current"=w1460:dbl)
                  }
                  frame Disabled {
                  }
                }
                n327 = case shown="\"HapticBump\"" w1128 {
                  tunnel: w1133 -> [w1151 w1275 _ _ _ w1360 w1401 w1433]
                  tunnel: w1138 -> [w1156 w1265 w1283 w1299 w1331 w1357 w1376 w1440]
                  tunnel: [w1155 w1270 w1288 w1302 w1330 w1364 w1407 w1431] -> w1137
                  tunnel: [w1154 w1273 w1290 w1304 w1334 w1366 w1410 w1441] -> w1136
                  tunnel: [w1153 w1271 w1284 w1300 w1313 w1358 w1391 w1429] -> w1130
                  tunnel: [w1150 TRUE ("profile complete?") TRUE ("profile complete?") TRUE ("profile complete?") w1342 TRUE ("profile complete?") TRUE ("profile complete?") w1426] -> w1134
                  tunnel: [w1152 0.0 ("u") 0.0 ("u") 0.0 ("u") w1320 0.0 ("u") 0.0 ("u") w1427] -> w1123
                  tunnel: w1126 -> [w1149 _ _ _ w1322 _ _ w1420]
                  tunnel: w1127 -> [w1148 w1264 w1282 w1298 w1344 w1356 w1375 w1419]
                  tunnel: w1124 -> [_ _ _ _ w1336 _ _ _]
                  tunnel: [w1147 w1262 w1280 w1296 w1312 w1354 w1372 w1417] -> w1122
                  tunnel: w1121 -> [w1147 w1262 w1280 w1296 w1321 w1354 w1372 w1417]
                  frame "RangeOfMotion" {
                    n328 = local read "ROM State"() -> (w1157:T3)
                    n329 = case shown="\"AutomaticPassive\"" w1157 {
                      selector: w1157 -> [w1169 _]
                      tunnel: [TRUE ("profile complete?") w1216] -> w1150
                      tunnel: w1156 -> [w1165 w1217]
                      tunnel: [w1170 w1215] -> w1155
                      tunnel: [FALSE w1214] -> w1154
                      tunnel: [w1172 w1214] -> w1153
                      tunnel: [0.0 ("u") w1218] -> w1152
                      tunnel: w1151 -> [w1167 w1213]
                      tunnel: w1149 -> [w1162 w1211]
                      tunnel: w1148 -> [w1159 w1210]
                      frame "Active", "Passive" {
                        n330 = Unbundle By Name(w1162) -> ("Position [deg]"=w1161:dbl)
                        n331 = Equal?(x=w1165, y=i16 1) -> (x = y?=w1166:bool)
                        n332 = Equal To 0?(x=w1167) -> (x = 0?=w1168:bool)
                        n333 = Unbundle By Name(w1159) -> ("Phase Trial Count"=w1160:i16)
                        n334 = local read "StartSignal"() -> (w1175:bool)
                        n335 = And "first passive iteration?"(x=w1166, y=w1168) -> (x .and. y?=w1163:bool)
                        n336 = case shown="True" w1175 {
                          tunnel: w1165 -> [w1193 w1194]
                          tunnel: [FALSE TRUE] -> w1172
                          tunnel: [w1193 w1196] -> w1170
                          tunnel: w1169 -> [_ w1197]
                          tunnel: w1160 -> [_ w1195]
                          frame False {
                            # "Ongoing trial"
                          }
                          frame True {
                            # "User finished trial, switch to next subtask if this was 3rd trial"
                            n337 = Equal?(x=w1194, y=w1195) -> (x = y?=w1199:bool)
                            n338 = case shown="True" w1199 {
                              tunnel: w1197 -> [_ w1205]
                              tunnel: w1194 -> [w1201 _]
                              tunnel: [w1200 i16 1] -> w1196
                              frame False {
                                n339 = Increment(x=w1201) -> (x+1=w1200:i16)
                              }
                              frame True {
                                n340 = case shown="\"Passive\"" w1205 {
                                selector: w1205 -> [_ _ w1208]
                                tunnel: [ROM_States."Passive" ("ROM State") ROM_States."AutomaticPassive" ("ROM State") w1208] -> w1204
                                frame "Active" {
                                }
                                frame "Passive" {
                                }
                                frame "AutomaticPassive" {
                                }
                                }
                                n341 = local write "StartSignal"(FALSE ("StartSignal")) -> ()
                                n342 = local write "ROM State"(w1204) -> ()
                              }
                            }
                          }
                        }
                        n343 = Unbundle By Name(w1159) -> ("Left Hand"=w1158:bool)
                        n344 = case "Calculate ROM during passive motion" shown="\"Passive\"" w1169 {
                          tunnel: w1161 -> [_ w1181]
                          tunnel: w1158 -> [_ w1177]
                          tunnel: w1163 -> [_ w1176]
                          frame Default {
                          }
                          frame "Passive" {
                            n345 = case shown="False" w1176 {
                              tunnel: w1181 -> [w1190 w1191]
                              tunnel: [w1190 w1191] -> w1180
                              tunnel: [w1189 w1191] -> w1179
                              tunnel: [w1188 w1191] -> w1178
                              frame False {
                                n346 = local read "ROM max"() -> (w1189:dbl)
                                n347 = local read "ROM min"() -> (w1188:dbl)
                              }
                              frame True {
                                "ROM max" <- w1191
                                "ROM min" <- w1191
                              }
                            }
                            n348 = Max & Min(x=w1179, y=w1180) -> (max(x,y)=w1185:dbl, min(x,y)=w1186:dbl)
                            n349 = Max & Min(x=w1180, y=w1178) -> (max(x,y)=w1182:dbl, min(x,y)=w1183:dbl)
                            n350 = Select(t=w1185, s=w1177, f=w1186) -> (s? t:f=w1187:dbl)
                            n351 = Select(t=w1183, s=w1177, f=w1182) -> (s? t:f=w1184:dbl)
                            n352 = local write "ROM max"(w1187) -> ()
                            n353 = local write "ROM min"(w1184) -> ()
                          }
                        }
                      }
                      frame "AutomaticPassive" {
                        # "Generates a sinewave with the determined max range of motion"
                        n354 = Equal To 0?(x=w1213) -> (x = 0?=w1212:bool)
                        n355 = flat-sequence "Calculate and execute sinewave" {
                          tunnel: [w1232] -> w1218
                          tunnel: [w1229] -> w1216
                          tunnel: w1212 -> [w1226]
                          tunnel: w1211 -> [w1224]
                          tunnel: w1210 -> [w1220]
                          frame #0 {
                            n356 = feedback #7() -> (w1231:cluster{"time (s)":dbl, "setpoint":dbl}[])  [unwired: 1 in]
                            n357 = case shown="True" w1226 {
                              tunnel: [w1233 w1248] -> w1230
                              tunnel: w1231 -> [w1233 _]
                              tunnel: w1220 -> [_ w1235]
                              frame False {
                              }
                              frame True {
                                # "Sine wave amplitude"
                                # "2s movement \n(1s between flexion \n& extension)"
                                n358 = local read "ROM max"() -> (w1243:dbl)
                                n359 = local read "ROM min"() -> (w1239:dbl)
                                n360 = Unbundle By Name(w1235) -> ("Left Hand"=w1234:bool)
                                n361 = Subtract(x=w1243, y=w1239) -> (x-y=w1241:dbl)
                                n362 = Absolute Value(x=w1241) -> (abs(x)=w1242:dbl)
                                n363 = Divide(x=w1242, y=2.0) -> (x/y=w1236:dbl)
                                n364 = local read "Zero Position"() -> (w1245:dbl)
                                n365 = Negate(x=w1236) -> (-x=w1238:dbl)
                                n366 = Select(t=w1236, s=w1234, f=w1238) -> (s? t:f=w1237:dbl)
                                n367 = call "Sine_Trajectory.vi"("Amplitude"=w1237, "Middle Position"=w1245, "Frequency (Hz)"=1.0, "Duration (s)"=2.0, "Sampling Period (s)"=0.001 ("Period (s)")) -> ("Profile"=w1248:cluster{"time (s)":dbl, "setpoint":dbl}[])  [unwired: 6 in]
                              }
                            }
                            n368 = feedback-in #7(w1230) -> ()
                            n369 = Unbundle By Name(w1224) -> ("Position [deg]"=w1223:dbl, "Velocity [deg/s]"=w1222:dbl, "Control Loop Period [s]"=w1221:dbl)
                            n370 = feedback #8() -> (w1227:bool)  [unwired: 1 in]
                            n371 = Or(x=w1226, y=w1227) -> (x .or. y?=w1228:bool)
                            n372 = call "sine_params.vi"() -> ("PID Settings"=w1219:T44)  [unwired: 19 in]
                            n373 = call <vilib>:"PID Setpoint Profile.vi"("reinitialize? (F)"=w1228, "setpoint profile"=w1230) -> ("profile complete?"=w1229:bool, "setpoint"=w1225:dbl)  [unwired: 4 in, 2 out]
                            n374 = feedback-in #8(w1229) -> ()
                            n375 = call "ENPID.vi"("PID Settings"=w1219, "r"=w1225, "y"=w1223, "dy/dt"=w1222, "dt (s)"=w1221) -> ("u"=w1232:dbl)  [unwired: 13 in, 1 out]
                          }
                        }
                        n376 = Unbundle By Name(w1210) -> ("Phase Trial Count"=w1209:i16)
                        n377 = case shown="True" w1216 {
                          tunnel: w1217 -> [w1250 w1252]
                          tunnel: [w1250 w1254] -> w1215
                          tunnel: [FALSE w1253] -> w1214
                          tunnel: w1209 -> [_ w1251]
                          frame False {
                          }
                          frame True {
                            n378 = Equal?(x=w1252, y=w1251) -> (x = y?=w1255:bool)
                            n379 = case "Finish up Task" shown="True" w1255 {
                              tunnel: [w1256 i16 0 ("Trial Nr")] -> w1254
                              tunnel: w1252 -> [w1257 _]
                              tunnel: [FALSE TRUE] -> w1253
                              frame False {
                                n380 = Increment(x=w1257) -> (x+1=w1256:i16)
                              }
                              frame True {
                                n381 = local write "StartSignal"(FALSE) -> ()
                              }
                            }
                          }
                        }
                      }
                    }
                  }
                  frame "Force" {
                    # "Increment TrialNr\nif cycles reached and not last trial"
                    # "Finish Trial after the\nset amount of cycles"
                    n382 = Unbundle By Name(w1264) -> ("Phase Trial Count"=w1263:i16)
                    n383 = Multiply(x=w1263, y=i16 2) -> (x*y=w1266:i16)
                    n384 = Equal?(x=w1265, y=w1266) -> (x = y?=w1273:bool)
                    n385 = Equal?(x=w1275, y=3000) -> (x = y?=w1271:bool)
                    n386 = Not(x=w1273) -> (.not. x?=w1272:bool)
                    n387 = And(x=w1272, y=w1271) -> (x .and. y?=w1269:bool)
                    n388 = case "Trial Increment" shown="True" w1269 {
                      tunnel: w1265 -> [w1277 w1279]
                      tunnel: [w1277 w1278] -> w1270
                      frame False {
                      }
                      frame True {
                        n389 = Increment(x=w1279) -> (x+1=w1278:i16)
                      }
                    }
                  }
                  frame "PreciseReaching" {
                    # "Trial Finished"
                    # "Increment Trial Count\nif cycles reached and not last trial"
                    # "Finish Trial once we get another\nstart signal"
                    n390 = Unbundle By Name(w1282) -> ("Phase Trial Count"=w1281:i16)
                    n391 = Multiply(x=i16 2, y=w1281) -> (x*y=w1286:i16)
                    n392 = local read "StartSignal"() -> (w1284:bool)
                    n393 = Equal? "Max Trials Reached"(x=w1283, y=w1286) -> (x = y?=w1290:bool)
                    n394 = Not(x=w1290) -> (.not. x?=w1289:bool)
                    n395 = And(x=w1289, y=w1284) -> (x .and. y?=w1287:bool)
                    n396 = case "Trial Increment" shown="True" w1287 {
                      tunnel: w1283 -> [w1293 w1295]
                      tunnel: [w1293 w1294] -> w1288
                      frame False {
                      }
                      frame True {
                        n397 = Increment(x=w1295) -> (x+1=w1294:i16)
                      }
                    }
                  }
                  frame "ActiveMatching", "TeachAndReproduce" {
                    # "Trial Finished"
                    # "Increment Trial Count\nif cycles reached and not last trial"
                    # "Finish Trial once we get another\nstart signal"
                    n398 = Unbundle By Name(w1298) -> ("Phase Trial Count"=w1297:i16)
                    n399 = local read "StartSignal"() -> (w1300:bool)
                    n400 = Equal? "Max Trials Reached"(x=w1299, y=w1297) -> (x = y?=w1304:bool)
                    n401 = Not(x=w1304) -> (.not. x?=w1303:bool)
                    n402 = And(x=w1303, y=w1300) -> (x .and. y?=w1301:bool)
                    n403 = case "Trial Increment" shown="True" w1301 {
                      tunnel: w1299 -> [w1307 w1309]
                      tunnel: [w1307 w1308] -> w1302
                      frame False {
                      }
                      frame True {
                        n404 = Increment(x=w1309) -> (x+1=w1308:i16)
                      }
                    }
                  }
                  frame "HapticBump" {
                    # "this is to put direction to 0 at end of each trial"
                    # "handle direction"
                    # "do force/torque"
                    # "here we check if we are in range of haptic bump"
                    # "invert the current depending on direction\n(have to multiply by -1 as u have defined direction -1 going from 0°-(-125°)"
                    # "This is direction indication\nIf -1 means down if 1 up"
                    # "Current for gravity compensation"
                    # "Trial Finished"
                    # "Increment Trial Count\nif cycles reached and not last trial"
                    # "Finish Trial once we get another\nstart signal"
                    n405 = Unbundle By Name(w1344) -> ("Phase Trial Count"=w1345:i16)
                    n406 = local read "Plateau length [deg]"() -> (w1338:dbl)
                    n407 = local read "Ramp length [deg]"() -> (w1337:dbl)
                    n408 = local read "Haptic Bump Force [N]"() -> (w1335:dbl)
                    n409 = Unbundle By Name(w1322) -> ("Position [deg]"=w1324:dbl)
                    n410 = local read "Target Position [deg]"() -> (w1326:dbl)
                    n411 = Divide(x=w1338, y=2.0) -> (x/y=w1340:dbl)
                    n412 = Equal?(x=w1321, y=0.0) -> (x = y?=w1327:bool)
                    n413 = Add(x=w1340, y=w1337) -> (x+y=w1323:dbl)
                    n414 = Subtract(x=w1326, y=w1324) -> (x-y=w1333:dbl)
                    n415 = Absolute Value(x=w1333) -> (abs(x)=w1343:dbl)
                    n416 = local read "StartSignal"() -> (w1313:bool)
                    n417 = Equal? "Max Trials Reached"(x=w1331, y=w1345) -> (x = y?=w1334:bool)
                    n418 = Not(x=w1334) -> (.not. x?=w1332:bool)
                    n419 = In Range and Coerce(upper limit=w1323, x=w1343, lower limit=0.0) -> (In Range?=w1342:bool)  [unwired: 1 out]
                    n420 = local read "Starting position"() -> (w1314:dbl)
                    n421 = And(x=w1332, y=w1313) -> (x .and. y?=w1346:bool)
                    n422 = call "RampUp.vi"("Target Position [deg]"=w1326, "Haptic Bump Force [N]"=w1335, "Position [deg]"=w1324, "Are we within haptic bump range?"=w1342, "Plateau length"=w1338, "Ramp length"=w1337) -> ("CurrentOut [A]"=w1317:dbl)  [unwired: 13 in]
                    n423 = case "Trial Increment" shown="True" w1346 {
                      tunnel: w1331 -> [w1351 w1353]
                      tunnel: [w1351 w1352] -> w1330
                      frame False {
                      }
                      frame True {
                        n424 = Increment(x=w1353) -> (x+1=w1352:i16)
                      }
                    }
                    n425 = Not Equal?(x=w1331, y=w1330) -> (x != y?=w1329:bool)
                    n426 = Or(x=w1327, y=w1329) -> (x .or. y?=w1328:bool)
                    n427 = call "InvertDirection.vi"("did we just start?"=w1328, "Numeric 3"=w1321, "Target Position [deg]"=w1326, "Position [deg]"=w1324, "Starting position"=w1314, "HalfOfHapticBumpLength"=w1323) -> ("Numeric"=w1311:dbl, "start value"=→"start value":dbl, "difference at start"=→"difference at start":dbl)  [unwired: 1 in, 6 out]
                    n428 = case shown="True" w1313 {
                      tunnel: w1311 -> [w1347 w1349]
                      tunnel: [w1347 w1348] -> w1312
                      frame False {
                      }
                      frame True {
                        n429 = Multiply(x=0.0, y=w1349) -> (x*y=w1348:dbl)
                      }
                    }
                    "Direction" <- w1312
                    n430 = Multiply(x=w1312, y=-1.0) -> (x*y=w1318:dbl)
                    n431 = Multiply(x=w1317, y=w1318) -> (x*y=w1316:dbl)
                    n432 = Add(x=w1316, y=w1336) -> (x+y=w1320:dbl)
                  }
                  frame "Motor", Default {
                    # "Trial Finished"
                    # "Increment Trial Count\nif cycles reached and not last trial"
                    # "Finish Trial after 4 seconds"
                    n433 = Unbundle By Name(w1356) -> ("Phase Trial Count"=w1355:i16)
                    n434 = Greater Or Equal?(x=w1360, y=4000) -> (x >= y?=w1358:bool)
                    n435 = Multiply(x=i16 2, y=w1355) -> (x*y=w1362:i16)
                    n436 = Equal? "Max Trials Reached"(x=w1357, y=w1362) -> (x = y?=w1366:bool)
                    n437 = Not(x=w1366) -> (.not. x?=w1365:bool)
                    n438 = And(x=w1365, y=w1358) -> (x .and. y?=w1363:bool)
                    n439 = case "Trial Increment" shown="True" w1363 {
                      tunnel: w1357 -> [w1369 w1371]
                      tunnel: [w1369 w1370] -> w1364
                      frame False {
                      }
                      frame True {
                        n440 = Increment(x=w1371) -> (x+1=w1370:i16)
                      }
                    }
                  }
                  frame "Sensorimotor" {
                    w1384 = 0.0008377580409572782  # (2*pi*4) / 30'000
                    w1383 = 0.0004188790204786391  # (2*pi*2) / 30'000
                    w1382 = 0.00020943951023931956  # (2*pi*1) / 30'000
                    # "Increment Trial when finished\nand not last trial"
                    n441 = Equal To 0?(x=w1401) -> (x = 0?=w1400:bool)
                    n442 = Unbundle By Name(w1375) -> ("Phase Trial Count"=w1373:i16, "Left Hand"=w1374:bool)
                    n443 = call "Tick Count3"() -> ("Tick Count(mSec)"=w1398:u32)
                    n444 = feedback #9() -> (w1399:u32)  [unwired: 1 in]
                    n445 = Select(t=w1398, s=w1400, f=w1399) -> (s? t:f=w1397:u32)
                    n446 = feedback-in #9(w1397) -> ()
                    n447 = Less Or Equal? "InSlowPhase"(x=w1376, y=w1373) -> (x <= y?=w1413:bool)
                    n448 = Subtract "ms since start"(x=w1398, y=w1397) -> (x-y=w1392:u32)
                    n449 = Select(t=u32 1, s=w1413, f=u32 3) -> (s? t:f=w1393:u32)
                    n450 = Greater Or Equal? "IsComplete?"(x=w1392, y=u32 30000) -> (x >= y?=w1391:bool)
                    n451 = Multiply "speedmul * t"(x=w1393, y=w1392) -> (x*y=w1386:u32)
                    n452 = To Double Precision Float(number=w1386) -> (double precision float=w1385:dbl)
                    n453 = Multiply(x=w1385, y=w1382) -> (x*y=w1389:dbl)
                    n454 = Multiply(x=w1385, y=w1383) -> (x*y=w1388:dbl)
                    n455 = Multiply(x=w1385, y=w1384) -> (x*y=w1387:dbl)
                    n456 = Sine(x=w1388) -> (sin(x)=w1405:dbl)
                    n457 = Sine(x=w1387) -> (sin(x)=w1403:dbl)
                    n458 = Sine(x=w1389) -> (sin(x)=w1406:dbl)
                    n459 = local read "Starting position"() -> (w1402:dbl)
                    n460 = Add(x=w1406, y=w1405) -> (x+y=w1404:dbl)
                    n461 = Select(t=15.0 ("x"), s=w1374, f=-15.0 ("x")) -> (s? t:f=w1377:dbl)
                    n462 = Multiply(x=i16 2 ("y"), y=w1373) -> (x*y=w1412:i16)
                    n463 = Add(x=w1404, y=w1403) -> (x+y=w1381:dbl)
                    n464 = Multiply(x=w1377, y=w1381) -> (x*y=w1380:dbl)
                    n465 = Add(x=w1380, y=w1402) -> (x+y=w1390:dbl)
                    n466 = Equal? "Max Trials Reached"(x=w1376, y=w1412) -> (x = y?=w1410:bool)
                    n467 = local write "Target Position [deg]"(w1390) -> ()
                    n468 = Not(x=w1410) -> (.not. x?=w1414:bool)
                    n469 = And(x=w1414, y=w1391) -> (x .and. y?=w1409:bool)
                    n470 = Increment(x=w1376) -> (x+1=w1408:i16)
                    n471 = Select(t=w1408, s=w1409, f=w1376) -> (s? t:f=w1407:i16)
                  }
                  frame "PositionMatching", "PassiveMatching" {
                    n472 = Equal To 0? "First Iteration"(x=w1433) -> (x = 0?=w1432:bool)
                    n473 = Unbundle By Name(w1420) -> ("Position [deg]"=w1421:dbl)
                    n474 = case "Check if first Iteration of Trial" shown="False" w1432 {
                      tunnel: [w1442 w1443] -> w1430
                      frame False {
                        n475 = local read "MovingToTarget"() -> (w1442:bool)
                      }
                      frame True {
                        w1443 = TRUE ("FirstRound")
                        "MovingToTarget" <- w1443
                      }
                    }
                    n476 = feedback #10() -> (w1439:cluster{"time (s)":dbl, "setpoint":dbl}[])  [unwired: 1 in]
                    n477 = feedback #11(TRUE ("profile complete?")) -> (w1436:bool)
                    n478 = Or(x=w1432, y=w1436) -> (x .or. y?=w1435:bool)
                    n479 = case shown="False" w1435 {
                      tunnel: [w1448 w1450] -> w1438
                      tunnel: w1439 -> [w1448 _]
                      tunnel: w1421 -> [_ w1451]
                      frame False {
                      }
                      frame True {
                        n480 = local read "Target Position [deg]"() -> (w1449:dbl)
                        n481 = call "motion_create_minimum_jerk.vi"("Initial Position"=w1451, "Final Position"=w1449, "Initial Time [s]"=0.0, "Final Time [s]"=3.0, "Delta Time [s]"=0.01) -> ("Profile"=w1450:cluster{"time (s)":dbl, "setpoint":dbl}[])  [unwired: 10 in]
                      }
                    }
                    n482 = feedback-in #10(w1438) -> ()
                    n483 = case "Deactivates StartSignal\nuntil moving is completed" shown="False" w1430 {
                      tunnel: [w1444 FALSE ("Boolean")] -> w1429
                      frame False {
                        # "StartSignal acts \nas finish signal"
                        n484 = local read "StartSignal"() -> (w1444:bool)
                      }
                      frame True {
                      }
                    }
                    n485 = Unbundle By Name(w1420) -> ("Position [deg]"=w1422:dbl, "Velocity [deg/s]"=w1423:dbl, "Control Loop Period [s]"=w1424:dbl)
                    n486 = call <vilib>:"PID Setpoint Profile.vi"("reinitialize? (F)"=w1435, "setpoint profile"=w1438) -> ("profile complete?"=w1426:bool, "setpoint"=w1425:dbl)  [unwired: 4 in, 2 out]
                    n487 = feedback-in #11(w1426) -> ()
                    n488 = call "min_jerk_params.vi"() -> ("PID Settings"=w1428:T44)  [unwired: 19 in]
                    n489 = call "ENPID.vi"("PID Settings"=w1428, "r"=w1425, "y"=w1422, "dy/dt"=w1423, "dt (s)"=w1424) -> ("u"=w1427:dbl)  [unwired: 13 in, 1 out]
                    n490 = And(x=w1430, y=w1426) -> (x .and. y?=w1434:bool)
                    n491 = case "Finish Trial" shown="False" w1429 {
                      tunnel: w1440 -> [w1455 w1458]
                      tunnel: [w1455 w1457] -> w1431
                      frame False {
                      }
                      frame True {
                        n492 = Increment(x=w1458) -> (x+1=w1457:i16)
                        n493 = local write "Target state?"(FALSE ("TargetState")) -> ()
                      }
                    }
                    n494 = case "Start Probe" shown="True" w1434 {
                      frame False {
                      }
                      frame True {
                        n495 = local write "Target state?"(TRUE ("TargetState")) -> ()
                        n496 = local write "MovingToTarget"(FALSE ("FirstRound")) -> ()
                      }
                    }
                    n497 = Unbundle By Name(w1419) -> ("Phase Trial Count"=w1418:i16)
                    n498 = Greater?(x=w1431, y=w1418) -> (0:w1441:bool)
                  }
                }
                n499 = Increment(x=w1133) -> (x+1=w1132:i32)
                n500 = And(x=w1136, y=w1130) -> (x .and. y?=w1131:bool)
                n501 = case shown="True" w1131 {
                  tunnel: w1130 -> [w1139 _]
                  tunnel: [w1140 Main_States."Resetting" ("Task states")] -> w1125
                  frame False {
                    # "Task Running"
                    n502 = case shown="True" w1139 {
                      tunnel: [Main_States."Show target" ("Task states") Main_States."StartTrial" ("Task states")] -> w1140
                      frame False {
                        # "Trial Running"
                      }
                      frame True {
                        # "Trial Finished"
                        n503 = local write "Target state?"(FALSE ("Target state?")) -> ()
                        n504 = local write "SkipSignal"(FALSE ("SkipSignal")) -> ()
                      }
                    }
                  }
                  frame True {
                    # "Assessment Finished"
                    n505 = local write "TaskFinished"(TRUE ("AssessmentFinished")) -> ()
                  }
                }
                n506 = Select(t=w1123, s=w1134, f=w1124) -> (s? t:f=w1135:dbl)
              }
              frame "Resetting" {
                w1467 = FALSE ("Target state?")
                # "Clear Patient Data and reset other state"
                n507 = local write "FrontendStartedSignal"(w1467) -> ()
                n508 = local write "SkipSignal"(w1467) -> ()
                n509 = local write "Target state?"(w1467) -> ()
                n510 = local write "SelectedHand"(Hand."None" ("SelectedHand")) -> ()
                n511 = local write "Starting Position Frontend [deg]"(0.0 ("Target Position Frontend [deg]")) -> ()
                n512 = local write "Target Position Frontend [deg]"(0.0 ("Target Position Frontend [deg]")) -> ()
                n513 = local write "Haptic Bump Force Frontend [N]"(0.0) -> ()
                n514 = local write "ROM State"(ROM_States."Active" ("ROM State")) -> ()
              }
              frame "WaitingForRestart" {
                # "Current Machine State"
                n515 = local read "RestartSignal"() -> (w1477:bool)
                n516 = local read "LogFileOpen"() -> (w1479:bool)
                n517 = Not(x=w1479) -> (.not. x?=w1478:bool)
                n518 = And(x=w1477, y=w1478) -> (x .and. y?=w1476:bool)
                n519 = case shown="True" w1476 {
                  tunnel: w1475 -> [w1483 _]
                  tunnel: [w1483 Main_States."Hand choice" ("Task states")] -> w1474
                  frame False {
                    # "Waiting for restart"
                  }
                  frame True {
                    # "Restart State Machine"
                    n520 = flat-sequence {
                      tunnel: FALSE ("Target state?") -> [w1487]
                      tunnel: [w1487] -> w1484
                      frame #0 {
                        n521 = local write "TaskFinished"(w1487) -> ()
                      }
                    }
                    n522 = local write "RestartSignal"(w1484) -> ()
                  }
                }
              }
            }
          }
          frame #4 {
            # "Robot State"
            # "Task Info"
            # "Machine State"
            # "Trial Nr"
            # "Loop count"
            # "Motor Current Setpoint"
            # "Send Motor Command"
            n523 = Unbundle By Name(w1491) -> ("Position [deg]"=w1494:dbl)
            n524 = call "TF_MotorCurrentOutput.vi"("Motor Current Setpoint [A]"=w1492) -> ("Motor Current Setpoint [V]"=w1505:dbl)
            n525 = local read "RestartSignal"() -> (w1497:bool)
            n526 = Not Equal?(x=Main_States."WaitingForRestart" ("Task states"), y=w1499) -> (x != y?=w1498:bool)
            n527 = And(x=w1498, y=w1497) -> (x .and. y?=w1496:bool)
            n528 = local read "StopSignal"() -> (w1502:bool)
            n529 = case "Initiate restart procedure" shown="True" w1496 {
              tunnel: w1499 -> [w1509 _]
              tunnel: [w1509 Main_States."Resetting" ("t")] -> w1495
              frame False {
              }
              frame True {
              }
            }
            "Machine State" <- w1495
            n530 = call "ConstrainOutput.vi"("Position [deg]"=w1494, "Motor Current Setpoint [V]"=w1505) -> ("Motor Output"=w1489:dbl)  [unwired: 9 in]
            n531 = Or(x="stop", y=w1502) -> (x .or. y?=w1504:bool)
            "StopRequested" <- w1504
            n532 = Build Array(w1489) -> (w1508:dbl[])
            n533 = call <vilib>:"Write.vi"("Values"=w1508, "AO Ref In"=w1490) -> ("AO Ref Out"=w1507:T24)  [unwired: 7 in, 1 out]
            "Current Setpoint [A]" <- w1492
            "Trial Nr" <- w1501
          }
        }
        n534 = node-c288() -> ()  [unwired: 1 in, 1 out]
      }
      n535 = node-c288(w245) -> ()  [unwired: 1 out]
      n536 = node-c288(w239) -> ()  [unwired: 1 out]
      n537 = node-c288(60 ("Priority"), 1 ("Processor")) -> (w231:T12)  [unwired: 2 in]
      n538 = timed-sequence {
        timing: w231 -> [_]
        timing-out: [_] -> w230
        tunnel: w219 -> [w255]
        tunnel: w227 -> [w254]
        n539 = timed-flat-sequence {
          tunnel: w255 -> [w262]
          tunnel: w254 -> [w257]
          # "NewPatient Event Notifier"
          # "Buffer"
          # "Index"
          # "TDMS File"
          # "PatientData"
          # "GroupName"
          # "TDMS Logging"
          n540 = node-c288() -> ()  [unwired: 1 in, 1 out]
          n541 = local read "Largest USB Partition Path"() -> (w256:path)
          n542 = Initialize Array(0.0 ("element"), 50 ("dimension size"), 14 ("dimension size")) -> (w261:dbl[][])
          n543 = while {
            shift-right: [w284] -> _
            shift-left: TypeDef_TDMS_States."WaitingForCreate" ("TDMS States") -> [w283]
            shift-right: [w282] -> _
            shift-left: _ -> [w281]
            shift-right: [w280] -> _
            shift-left: _ -> [w279]
            shift-right: [w276] -> _
            shift-left: _ -> [w278]
            tunnel: w256 -> [w277]
            shift-right: [w273] -> _
            shift-left: string[] ["Time [s]", "Position [deg]", "Target Position [deg]", "Target state?", "Frontend Started", "Trial Nr", "Velocity [deg/s]", "Current [A]", "Starting position [deg]", "Voltage force [V]", "Force [N]", "Force filtered [N] ", "Velocity unfiltered", "ROM State 0-Active 1-Passive 2-Automatic", "Haptic Bump Force  [N]"] -> [w275]
            tunnel: w262 -> [w272]
            shift-right: [w271] -> _
            shift-left: _ -> [w270]
            shift-right: [w268] -> _
            shift-left: w261 -> [w269]
            shift-right: [w267] -> _
            shift-left: _ -> [w266]
            tunnel: w257 -> [w265]
            stop <- w274 stop-if-true
            # "Stop when stop\nsignal is on\nand we are \nin a safe state"
            # "Logging"
            n544 = case shown="\"WaitingForCreate\"" w283 {
              selector: w283 -> [w290 _ w370 _ _ _]
              tunnel: [w288 w318 w385 TypeDef_TDMS_States."Close" ("TDMS States") w417 TypeDef_TDMS_States."WaitingForCreate" ("TDMS States")] -> w284
              tunnel: [w293 FALSE ("Button :: Stop") FALSE ("StopRequested") FALSE ("StopRequested") FALSE ("Button :: Stop") w438] -> w274
              tunnel: [w285 w306 w390 w402 w408 w436] -> w282
              tunnel: w281 -> [_ w310 w391 w403 w422 _]
              tunnel: [w294 w321 w392 w404 w421 _] -> w280
              tunnel: w279 -> [w294 _ w392 w404 w423 w441]
              tunnel: w278 -> [w296 _ w394 w405 w415 w439]
              tunnel: w277 -> [_ w305 _ _ _ _]
              tunnel: [w296 w299 w394 w405 w415 w439] -> w276
              tunnel: w275 -> [w295 w300 w393 w401 w412 w435]
              tunnel: [w295 w300 w393 w401 w412 w435] -> w273
              tunnel: w272 -> [_ w311 w389 _ _ _]
              tunnel: [w291 0 w377 0 0 0] -> w271
              tunnel: w270 -> [w291 _ w379 w397 _ _]
              tunnel: w269 -> [w297 w316 w384 w398 w413 w433]
              tunnel: [w297 w316 w382 w398 w413 w433] -> w268
              tunnel: [w298 w312 w367 w406 w410 w432] -> w267
              tunnel: w266 -> [_ w312 w367 w406 w410 w432]
              tunnel: w265 -> [w287 _ _ _ _ w431]
              frame "WaitingForCreate" {
                n545 = Wait on Notification "NewPatientSubmitted Event"(notifier=w287, timeout in ms (-1)=1000) -> (notification=w298:T6, timed out?=w286:bool, error out=w285:errorcluster)  [unwired: 2 in, 1 out]
                n546 = Select(t=w290, s=w286, f=TypeDef_TDMS_States."Create" ("TDMS States")) -> (s? t:f=w288:T10)
                n547 = local read "StopRequested"() -> (w293:bool)
              }
              frame "Create" {
                # "Has to match description of frontend's TaskType enum"
                n548 = flat-sequence {
                  tunnel: w310 -> [w345]
                  tunnel: [w345] -> w309
                  frame #0 {
                    n549 = local write "LogFileOpen"(TRUE ("LogFileOpen")) -> ()
                  }
                }
                n550 = Unbundle By Name(w312) -> ("Timestamp"=w319:string, "Mode"=w320:T5, "StudyName"=w302:string, "Name"=w301:string, "Left"=w303:bool)
                n551 = Build Path(base path=w305, name or relative path=w302) -> (appended path=w304:path)
                n552 = case shown="\"Sensorimotor\"" w320 {
                  tunnel: ["Range Of Motion Task" ("name or relative path") "Force Task" ("name or relative path") "Precise Reaching Task" ("name or relative path") "Passive Matching Task" ("name or relative path") "Active Matching Task" ("name or relative path") "Teach & Reproduce Task" ("name or relative path") "HapticBump" "Motor Task" ("name or relative path") "Sensorimotor Task" ("name or relative path") "Position Matching Task" ("name or relative path")] -> w299
                  frame "RangeOfMotion" {
                  }
                  frame "Force" {
                  }
                  frame "PreciseReaching" {
                  }
                  frame "PassiveMatching" {
                  }
                  frame "ActiveMatching" {
                  }
                  frame "TeachAndReproduce" {
                  }
                  frame "HapticBump" {
                  }
                  frame "Motor", Default {
                  }
                  frame "Sensorimotor" {
                  }
                  frame "PositionMatching" {
                  }
                }
                n553 = while {
                  shift-right: [w348] -> _
                  shift-left: w311 -> [w349]
                  shift-right: [w347] -> w308
                  shift-left: w309 -> [w347]
                  stop <- w350 stop-if-true
                  # "Clear Stale Data"
                  n554 = RT FIFO Read(0:w349) -> (8:w348:refnum<k33>, 10:w350:bool)  [unwired: 3 in, 3 out]
                }
                n555 = Build Path(base path=w304, name or relative path=w301) -> (appended path=w335:path)
                n556 = Select(t="Left Hand" ("name or relative path"), s=w303, f="Right Hand" ("name or relative path")) -> (s? t:f=w333:string)
                n557 = Build Path(base path=w335, name or relative path=w299) -> (appended path=w334:path)
                n558 = Build Path(base path=w334, name or relative path=w333) -> (appended path=w324:path)
                n559 = call <vilib>:"Check if File or Folder Exists.vi"("error in (no error)"=w308, "path"=w324) -> ("error out"=w327:errorcluster, "file or folder exists?"=w325:bool, "dup path"=w326:path)  [unwired: 7 in]
                n560 = case shown="False" w325 {
                  tunnel: w326 -> [w354 w355]
                  tunnel: [w353 w356] -> w330
                  tunnel: w327 -> [w352 w356]
                  tunnel: [w351 w355] -> w332
                  frame False {
                    n561 = Create Folder(path (use dialog)=w354, error in=w352) -> (created path=w351:path, error out=w353:errorcluster)  [unwired: 1 in, 1 out]
                  }
                  frame True {
                  }
                }
                n562 = flat-sequence {
                  tunnel: [w344] -> w315
                  tunnel: w307 -> [w339]
                  tunnel: [w339] -> w306
                  frame #0 {
                    n563 = local read "TaskFinished"() -> (w340:bool)
                    n564 = local read "StopRequested"() -> (w343:bool)
                    n565 = local read "RestartSignal"() -> (w342:bool)
                    n566 = Or(x=w342, y=w343) -> (x .or. y?=w341:bool)
                    n567 = Or(x=w341, y=w340) -> (x .or. y?=w344:bool)
                  }
                }
                n568 = Concatenate Strings(w319, ".tdms") -> (w323:string)
                n569 = Build Path(base path=w332, name or relative path=w323) -> (appended path=w328:path)
                n570 = TDMS Open(7:enum16{"1.0", "2.0"}."2.0" ("file format version (2.0)"), 8:w330, 10:T11."create" ("operation (0:open)"), 11:w328) -> (0:w307:errorcluster, 3:w321:refnum<k34>)  [unwired: 3 in]
                n571 = Select(t=TypeDef_TDMS_States."Close" ("TDMS States"), s=w315, f=TypeDef_TDMS_States."Buffering" ("TDMS States")) -> (s? t:f=w318:T10)
              }
              frame "Buffering" {
                n572 = RT FIFO Read(0:w389, 2:10 ("timeout in ms (0)"), 3:w391) -> (9:w383:dbl[], 10:w380:bool, 11:w390:errorcluster)  [unwired: 1 in, 2 out]
                n573 = local read "TaskFinished"() -> (w375:bool)
                n574 = local read "StopRequested"() -> (w372:bool)
                n575 = local read "RestartSignal"() -> (w373:bool)
                n576 = Replace Array Subset(array=w384, new element=w383, index (row)=w379) -> (w382:dbl[][])  [unwired: 1 in]
                n577 = Or(x=w373, y=w372) -> (x .or. y?=w374:bool)
                n578 = Or(x=w374, y=w375) -> (x .or. y?=w371:bool)
                n579 = Select(t=TypeDef_TDMS_States."Flushing" ("TDMS States"), s=w371, f=w370) -> (s? t:f=w369:T10)
                n580 = Increment(x=w379) -> (x+1=w378:i32)
                n581 = Select(t=w379, s=w380, f=w378) -> (s? t:f=w377:i32)
                n582 = Equal?(x=50, y=w377) -> (x = y?=w387:bool)
                n583 = Select(t=TypeDef_TDMS_States."Write" ("TDMS States"), s=w387, f=w369) -> (s? t:f=w385:T10)
              }
              frame "Flushing" {
                n584 = Array Subset(array=w398, length (row)=w397) -> (w396:dbl[][])  [unwired: 3 in]
                n585 = TDMS Write(0:w404, 1:enum16{"decimated", "interleaved"}."interleaved" ("data layout (0:decimated)"), 5:w405, 7:w401, 9:w396, 11:w403) -> (15:w402:errorcluster)  [unwired: 3 out]
              }
              frame "Write" {
                n586 = TDMS Write(0:w423, 1:enum16{"decimated", "interleaved"}."interleaved" ("data layout (0:decimated)"), 5:w415, 7:w412, 9:w413, 11:w422) -> (4:w421:refnum<k34>, 15:w409:errorcluster)  [unwired: 2 out]
                n587 = flat-sequence {
                  tunnel: [w425] -> w414
                  tunnel: w409 -> [w424]
                  tunnel: [w424] -> w408
                  frame #0 {
                    n588 = local read "TaskFinished"() -> (w429:bool)
                    n589 = local read "StopRequested"() -> (w426:bool)
                    n590 = local read "RestartSignal"() -> (w427:bool)
                    n591 = Or(x=w427, y=w426) -> (x .or. y?=w428:bool)
                    n592 = Or(x=w428, y=w429) -> (x .or. y?=w425:bool)
                  }
                }
                n593 = Select(t=TypeDef_TDMS_States."Close" ("TDMS States"), s=w414, f=TypeDef_TDMS_States."Buffering" ("TDMS States")) -> (s? t:f=w417:T10)
              }
              frame "Close" {
                # "Ensure notifier buffer is empty before going back to WaitingForCreate"
                n594 = Cancel Notification(0:w431) -> (11:w430:errorcluster)  [unwired: 1 in, 2 out]
                n595 = TDMS Close(8:w430, 11:w441) -> (0:w437:errorcluster)  [unwired: 1 out]
                n596 = flat-sequence {
                  tunnel: w437 -> [w443]
                  tunnel: [w443] -> w436
                  frame #0 {
                    # "Unset after file was closed"
                    n597 = local write "LogFileOpen"(FALSE ("LogFileOpen")) -> ()
                  }
                }
                n598 = local read "StopRequested"() -> (w438:bool)
              }
            }
          }
          n599 = node-c288() -> ()  [unwired: 1 in, 1 out]
        }
      }
      n600 = node-c288(w230) -> ()  [unwired: 1 out]
      n601 = node-c288(w252) -> ()  [unwired: 1 out]
      n602 = Build Array(0.0) -> (w224:dbl[])
      n603 = call <vilib>:"Write.vi"("Values"=w224, "AO Ref In"=w226) -> ("AO Ref Out"=w225:T24)  [unwired: 7 in, 1 out]
      "Velocity_calib_value" <- w216
      "Force_calib_value" <- w222
    }
    frame #5 {
      # "Close sensor references"
      # "Close UDP Socket"
      # "Close TCP Listener"
      # "Reset"
      # "Force Sensor"
      # "Tachometer"
      # "Motor Current Monitor"
      # "Motor Current Setpoint"
      # "Encoder"
      # "Close everything"
      n604 = Unbundle By Name(w1525) -> ("Encoder"=w1524:T32, "Tachometer"=w1523:T34, "Motor Current Monitor"=w1522:T34, "Force Sensor"=w1521:T34)
      n605 = Release Notifier(notifier=w1528) -> ()  [unwired: 2 in, 3 out]
      n606 = TCP Close Connection(connection ID=w1531) -> (error out=w1529:errorcluster)  [unwired: 2 in, 1 out]
      n607 = UDP Close(connection ID=w1532) -> (error out=w1530:errorcluster)  [unwired: 1 in, 1 out]
      n608 = RT FIFO Delete(0:w1527) -> ()  [unwired: 2 in, 1 out]
      n609 = call <vilib>:"Close.vi"("AO Ref In"=w1533) -> ()  [unwired: 10 in, 1 out]
      n610 = call <vilib>:"Close.vi"("AO Ref In"=w1526) -> ()  [unwired: 10 in, 1 out]
      n611 = local write "UDP Error"(w1530) -> ()
      n612 = local write "TCP Error"(w1529) -> ()
      n613 = call <vilib>:"Stop.vi"("Encoder Ref In"=w1524) -> ("Encoder Ref Out"=w1534:T32)  [unwired: 9 in, 1 out]
      n614 = call <vilib>:"Close.vi"("AI Ref In"=w1523) -> ()  [unwired: 10 in, 1 out]
      n615 = call <vilib>:"Close.vi"("AI Ref In"=w1522) -> ()  [unwired: 10 in, 1 out]
      n616 = call <vilib>:"Close.vi"("AI Ref In"=w1521) -> ()  [unwired: 10 in, 1 out]
      n617 = call <vilib>:"Close.vi"("Encoder Ref In"=w1534) -> ()  [unwired: 10 in, 1 out]
    }
  }
